vi "主界面B010.vi"() -> ()   [LabVIEW 2013]
uses:
  <vilib>/Utility/file.llb/Read From Spreadsheet File (string).vi
  PCI8622_32.dll
panel:
  out "是否检测轴承":dbl
  out "KSJS":string
  in  "Y挡圈最大值":dbl
  in  "Y挡圈最小值":dbl
  in  "X挡圈最大值":dbl
  in  "X挡圈最小值":dbl
  in  "Y内圈最大值":dbl
  in  "Y内圈最小值":dbl
  in  "X内圈最大值":dbl
  in  "X内圈最小值":dbl
  in  "Y轴承最大值":dbl
  in  "Y轴承最小值":dbl format="%#_13g"
  in  "X轴承最大值":dbl=12.0 format="%#_13g"
  in  "X轴承最小值":dbl=1.0 format="%#_13g"
  out "员工ID":string
  out "压铆最大压力(N)":dbl
  out "压铆最小压力(N)":dbl
  out "3最大压装位移":dbl
  out "3最小压装位移":dbl
  out "3监控点":dbl
  in  "压轴承换向压力":dbl=5000.0
  out "换向指示1":bool
  in  "报警工步号":dbl
  out "报警提示":string
  in  "轴承压头速度（手动）":dbl
  in  "轴承压头位置（手动）":dbl
  in  "轴承内圈压头速度（手动）":dbl
  in  "轴承内圈压头位置（手动）":dbl
  out "换向指示2":bool
  in  "换向压力2":dbl=5000.0
  in  "工步号复位":bool
  out "通讯状态":bool
  in  "电动缸2ARST":bool
  in  "电动缸1ARST":bool
  out "内圈压头位置(mm)":dbl format="%#.1f"
  out "轴承压头位置(mm)":dbl format="%#.1f"
  out "型号数量":i32
  out "轴承压头位移(mm)":dbl format="%#.1f"
  out "内圈位移(mm)":dbl format="%#.1f"
  out "压铆位移(mm)":dbl format="%#.1f"
  out "压铆压力(N)":dbl format="%#.1f"
  out "error out 4":errorcluster
  out "error out 3":errorcluster
  out "error out 2":errorcluster
  out "ADODB._Connection Out":refnum<k7>
  out "error out":errorcluster
  out "B010本序不合格":bool
  out "内圈压力(N)":dbl format="%#.1f"
  out "轴承压头压力(N)":dbl format="%#.1f"
  out "B010本序合格":bool
  in  "停止":bool
  in  "自动工步号":dbl
  out "产品选型":dbl
  out "芯片ID":string
  out "自动操作状态":string
  in  "联线按钮":bool
  in  "选项卡控件":T1(tab)
  out "轴承区域最小压力(N)":dbl
  out "轴承区域最大压力(N)":dbl
  out "压轴承最大压力(N)":dbl
  out "轴承压装位移(mm)":dbl
  out "轴承最小压装位移(mm)":dbl
  out "轴承最大压装位移(mm)":dbl
  out "轴承监控点":dbl
  out "压装轴承，挡圈曲线":cluster{"Y":dbl[], "Y":dbl[]}[](graph) caption="压球涨堵头1"
  out "轴承最小压力(N)":dbl
  out "轴承最大压力(N)":dbl
  out "压装轴承合格":bool
  out "压装轴承不合格":bool
  out "轴承监控点压力(N)":dbl
  out "内圈区域压力最大值(N)":dbl
  out "内圈区域压力最小值(N)":dbl
  out "内圈压装最大压力(N)":dbl
  out "压装滚针轴承":cluster{"Y":dbl[], "Y":dbl[]}[](graph) caption="压球涨堵头1"
  out "压内圈不合格":bool
  out "压内圈合格":bool
  out "内圈最大压力(N)":dbl
  out "内圈最小压力(N)":dbl
  out "内圈监控点":dbl
  out "内圈最大压装位移(mm)":dbl
  out "内圈最小压装位移(mm)":dbl
  out "内圈实测压装位移(mm)":dbl
  out "内圈监控点压力(N)":dbl
  out "压铆区域内最大压力(N)":dbl
  out "压铆区域内最小压力(N)":dbl
  out "挡圈压铆":cluster{"Y":dbl[], "Y":dbl[]}[](graph) caption="压球涨堵头1"
  out "压挡圈合格":bool
  out "压挡圈不合格":bool
  out "压铆最大压力(N)":dbl
  out "压铆压装位移(mm)":dbl
  in  "轴承单步":bool
  in  "内圈单步":bool
  in  "挡圈单步":bool
  out "轴承正面":bool
  in  "伺服2P 启动":bool
  in  "伺服1P 启动":bool
  in  "快速上升速度":dbl
  in  "快速上升位置":dbl
  in  "慢速下降速度":dbl
  in  "慢速下降位置":dbl
  in  "快速下降速度":dbl
  in  "快速下降位置":dbl
  in  "快速上升速度":dbl
  in  "快速上升位置":dbl
  in  "慢速下降速度":dbl
  in  "慢速下降位置":dbl
  in  "快速下降速度":dbl
  in  "伺服2回零":bool
  in  "伺服2上升":bool
  in  "伺服2下降":bool
  in  "伺服2复位":bool
  in  "快速下降位置":dbl
  in  "伺服1回零":bool
  in  "伺服1上升":bool
  in  "伺服1下降":bool
  in  "伺服1复位":bool
  out "急停按钮":bool
  out "联线状态":bool
  out "光幕保护":bool
  out "气压报警":bool
  out "滑台右位":bool
  out "滑台左位":bool
  in  "滑台右移":bool
  in  "滑台左移":bool
  in  "增压缸下压":bool
  in  "增压缸上升":bool
  in  "增压缸增压":bool
  in  "增压缸卸压":bool
  in  "压铆压力零点偏移":dbl format="%#.2f"
  in  "压铆压力比例偏移":dbl format="%#.2f"
  in  "压铆位移零点偏移":dbl format="%#.2f"
  in  "压铆位移比例偏移":dbl format="%#.2f"
  in  "内圈压力零点偏移":dbl format="%#.2f"
  in  "内圈压力比例偏移":dbl format="%#.2f"
  in  "内圈位移零点偏移":dbl format="%#.2f"
  in  "内圈位移比例偏移":dbl format="%#.2f"
  in  "轴承压力零点偏移":dbl format="%#.2f"
  in  "轴承压力比例偏移":dbl format="%#.2f"
  in  "轴承位移零点偏移":dbl format="%#.2f"
  in  "轴承位移比例偏移":dbl format="%#.2f"
  in  "传感器参数查询":bool
  in  "传感器参数保存":bool
  in  "参数浏览表":string[][](table)=[["J709", "J728", "J706"], ["1", "1", "1"], ["168", "78.5", "98"], ["0", "500", "500"], ["10000", "5000", "5000"], ["0", "78", "97"], ["173", "80", "102"], ["183", "85.5", "79"], ["0", "500", "500"], ["20000", "5000", "5000"], ["0", "85.5", "83"], ["190", "86.5", "84"], ["250", "144", "194"], ["0", "55000", "55000"], ["100000", "65000", "65000"], ["0", "143", "143"], ["300", "147", "147"], ["-70", "-89\n", "-94"], ["20", "50", "50"], ["-80.95", "-104", "-113"], ["1", "1", "1"], ["0", "0", "0"], ["20", "50", "50"], ["-77", "-70", "-75"], ["20", "50", "50"], ["-92.5", "-82", "-87"], ["1", "1", "1"], ["0", "0", "0"], ["20", "50", "50"], ["1", "95", "97"], ["84", "96", "99"], ["2000", "500", "500"], ["4000", "5000", "5000"], ["81", "75", "79"], ["82", "77", "81"], ["0", "500", "500"], ["25000", "5000", "5000"], ["250", "184", "193"], ["252", "186", "194"], ["10000", "10000", "10000"], ["60000", "50000", "50000"], ["", "5000", "5000"], ["", "5000", "5000"], ["", "93", "93"], ["", "100", "102"], ["", "-10", "-10"], ["", "10000", "10000"], ["", "71", "77"], ["", "80", "85"], ["", "-10", "-10"], ["", "6000", "6000"], ["", "180", "190"], ["", "190", "197"], ["", "-10", "-10"], ["", "70000", "70000"], ["", "0", "1"]]
  in  "参数查询":bool
  in  "试验参数保存":bool
  in  "轴承区域最小位移(mm)":dbl=84.0
  in  "轴承区域最大位移(mm)":dbl=85.0
  in  "轴承区域最小压力(N)":dbl=500.0
  in  "轴承区域最大压力(N)":dbl=5000.0
  in  "内圈区域最小位移(mm)":dbl=90.0
  in  "内圈区域最大位移(mm)":dbl=91.0
  in  "内圈区域最小压力(N)":dbl=500.0
  in  "内圈区域最大压力(N)":dbl=5000.0
  in  "挡圈区域最小位移(mm)":dbl=250.0
  in  "挡圈区域最大位移(mm)":dbl=252.0
  in  "挡圈区域最小压力(N)":dbl=10000.0
  in  "挡圈区域最大压力(N)":dbl=60000.0
  out "员工姓名":string
  in  "型号选择":u16(ring)=1 items=["J709", "J728", "J706"]
  in  "参数加载":bool
  out "产品ID":string="0"
  # "判定参数"
  # "芜湖机械转向器装配线"
  # "齿轮轴总成装配"
  # "Q14070机械转向器装配线"
  # "湖北唯思凌科装备制造有限公司 设计开发 (C)2015"
  # "判定参数"
  # "实测值"
  # "判定参数"
  # "实测值"
  # "实测值"
  # "轴承\n压头\n设置"
  # "轴承\n内圈\n压头\n设置"
  # "传感器校验区"
  # "注意：\n具备权限的用户才能够修改传感器校验参数和试验参数！"
  # "关于传感器校验：\n1、传感器校验需要由具备资质的单位或部门进行校验。\n2、具备权限的用户才能够修改传感器校验参数和试验参数。\n3、修改校验参数方法：先将比例偏移置为1，修改零点偏移，使零点值与校验的传感器一致；然后根据增幅调整比例偏移。"
  # "注意：\n具备权限的用户才能够修改传感器校验参数和试验参数！"
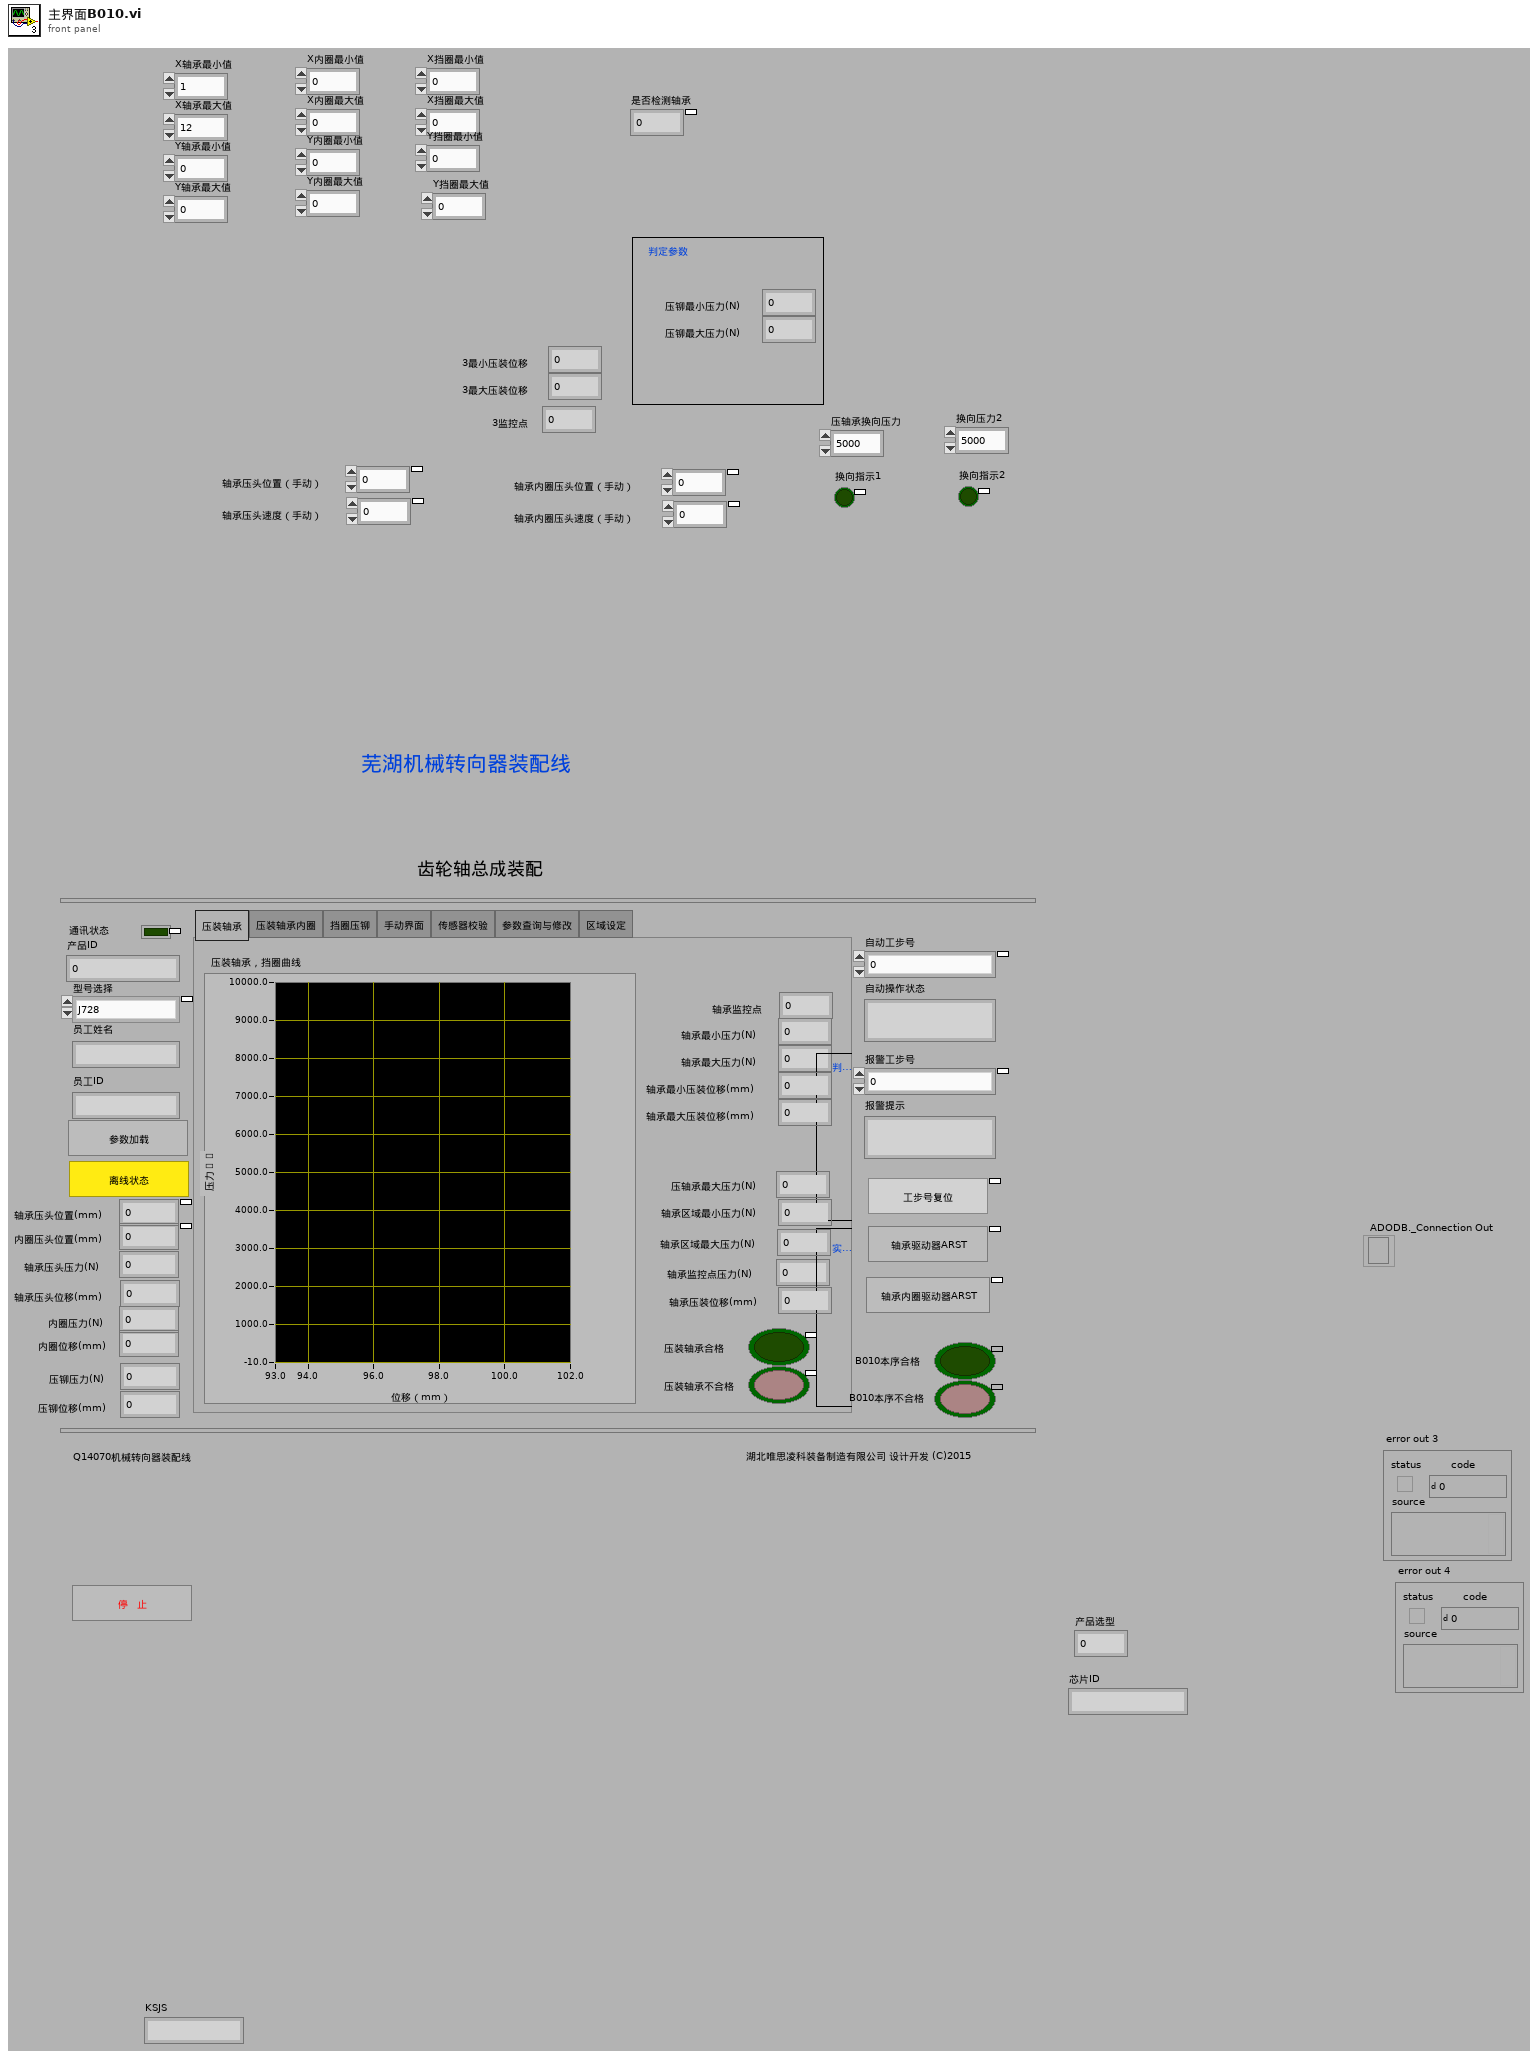
[diagram p1: front panel]
types:
  T1 = enum32{"压装轴承", "压装轴承内圈", "挡圈压铆", "手动界面", "传感器校验", "参数查询与修改", "区域设定"}
  T2 = typedef "imagedata.ctl" = cluster{"image type":i32, "image depth":i32, "image":u8[], "mask":u8[], "colors":u32[], "Rectangle":cluster{"left":i16, "top":i16, "right":i16, "bottom":i16}}
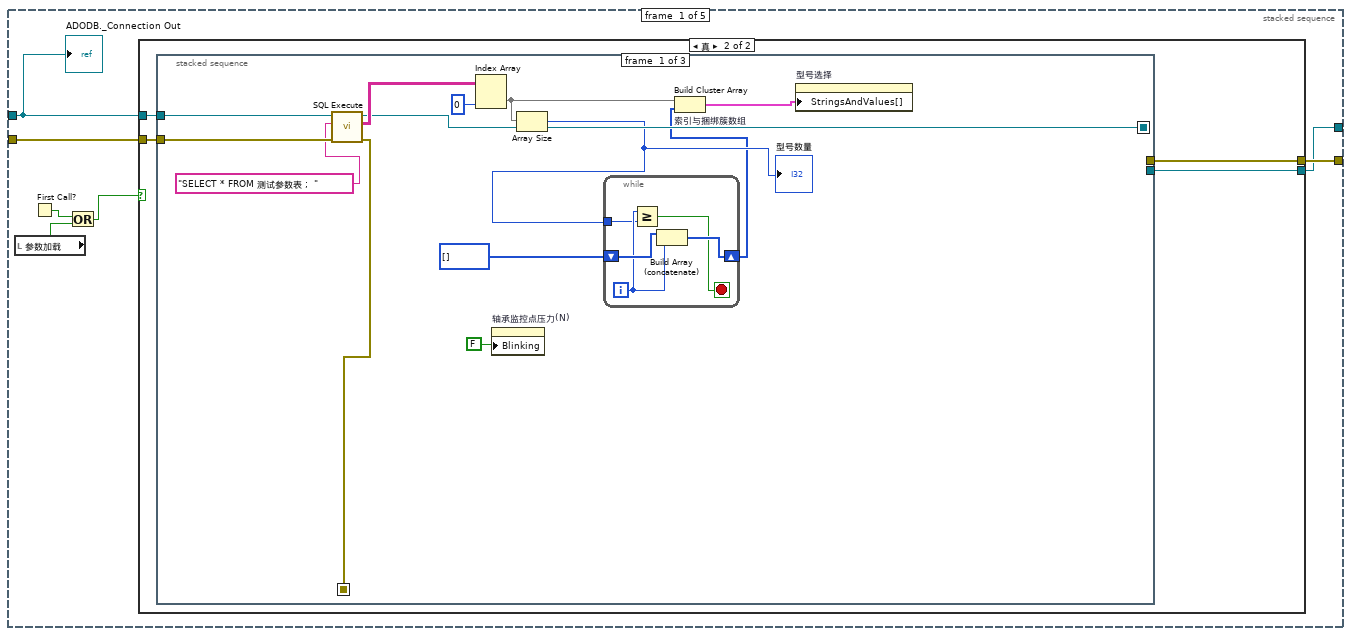
[diagram p2: hidden frame]
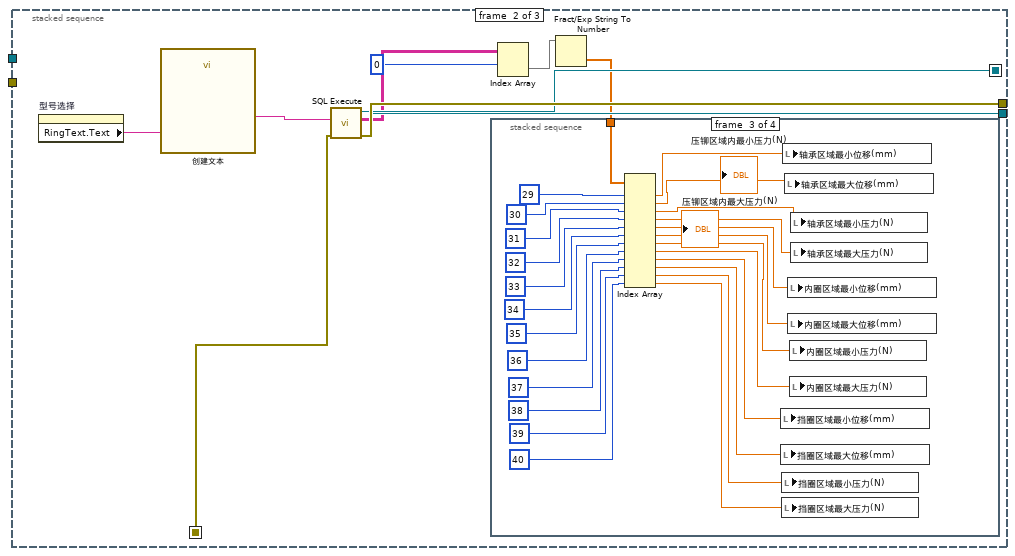
[diagram p4: hidden frame]
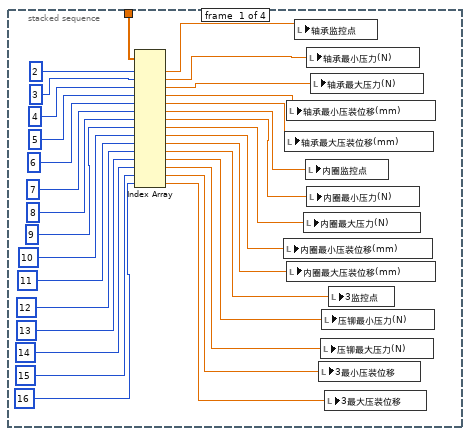
[diagram p5: hidden frame]
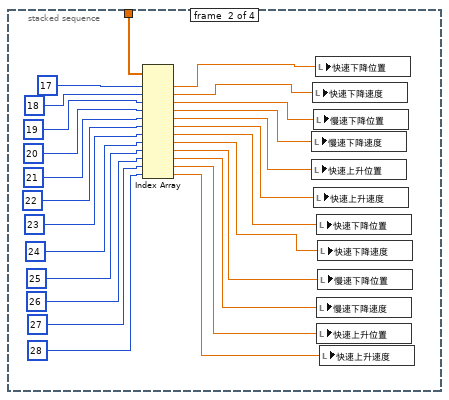
[diagram p6: hidden frame]
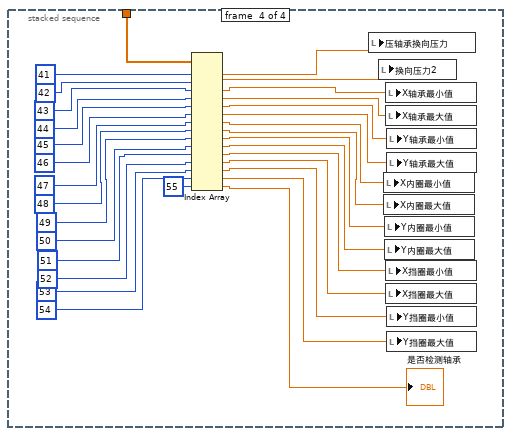
[diagram p7: hidden frame]
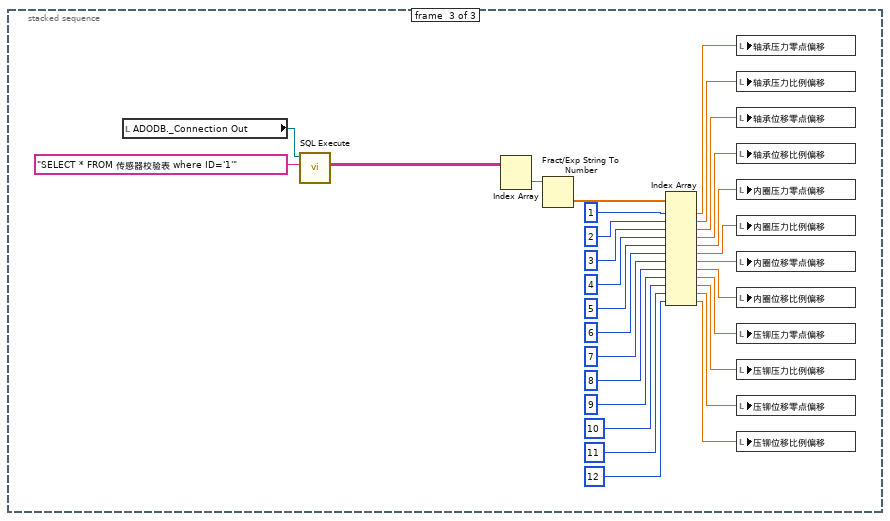
[diagram p8: hidden frame]
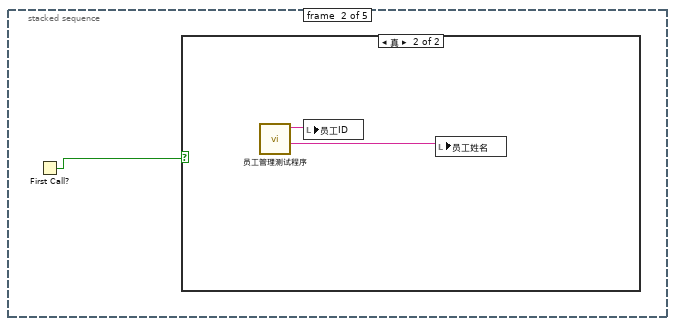
[diagram p9: hidden frame]
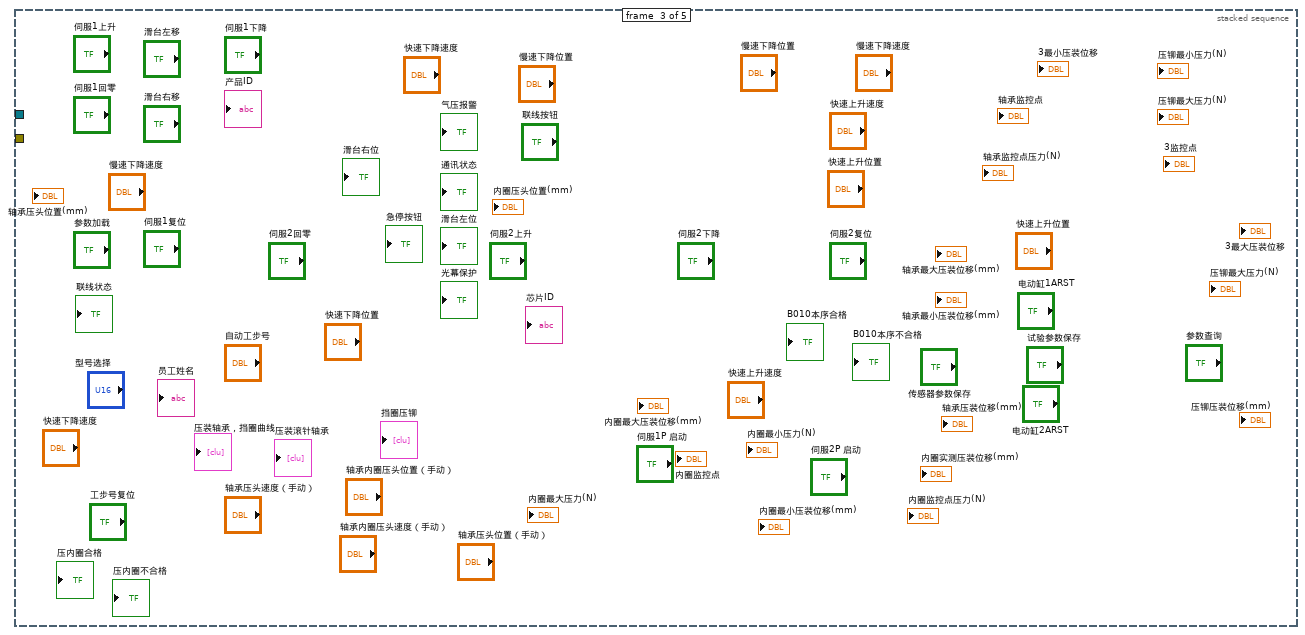
[diagram p11: hidden frame]
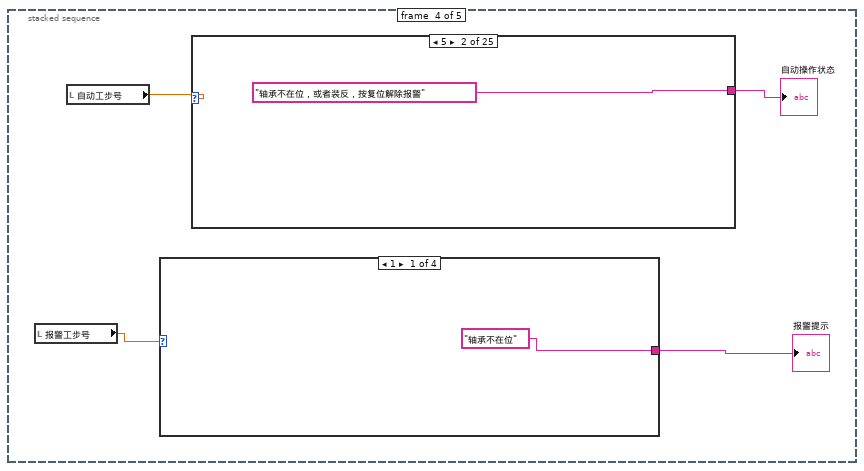
[diagram p12: hidden frame]
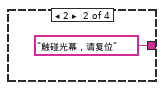
[diagram p13: hidden frame]
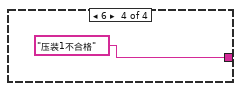
[diagram p15: hidden frame]
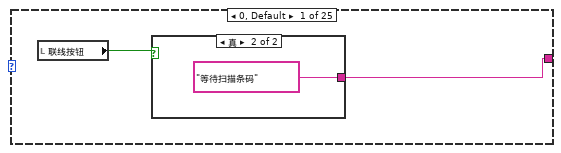
[diagram p16: hidden frame]
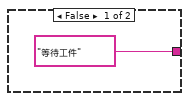
[diagram p17: hidden frame]
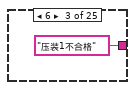
[diagram p18: hidden frame]
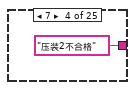
[diagram p19: hidden frame]
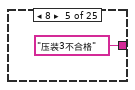
[diagram p20: hidden frame]
diagram:
  n1 = while {
    stop <- w10 stop-if-true
    n2 = local read "自动工步号"() -> (w8:dbl)
    n3 = Wait Until Next ms Multiple(millisecond multiple=u32 100 ("毫秒倍数")) -> ()  [unwired: 1 out]
    n4 = case shown="11" w8 {
      frame 0, Default {
      }
      frame 11 {
        n5 = flat-sequence {
          tunnel: [w27] -> w16
          tunnel: [w35] -> w22
          tunnel: [w34] -> w21
          tunnel: w16 -> [w33]
          tunnel: w22 -> [w61]
          tunnel: w21 -> [w59]
          tunnel: [w67] -> w20
          tunnel: [w66] -> w19
          tunnel: [w60] -> w14
          tunnel: w20 -> [w75]
          tunnel: w19 -> [w80]
          tunnel: [w77] -> w18
          tunnel: [w73] -> w17
          tunnel: [w72] -> w15
          tunnel: w14 -> [w72]
          tunnel: [w71] -> w13
          tunnel: [w70] -> w12
          tunnel: w18 -> [w89]
          tunnel: w17 -> [w88]
          tunnel: w15 -> [w85]
          tunnel: w13 -> [w87]
          tunnel: w12 -> [w86]
          tunnel: [w81] -> w11
          tunnel: w11 -> [w91]
          frame #0 {
            w25 = FALSE ("换向指示1")
            w32 = FALSE
            n6 = local write "压装轴承不合格"(w32) -> ()
            n7 = local write "压装轴承合格"(w32) -> ()
            n8 = Format Date/Time String(time format string (%c)="%Y%m%d%H%M%S" ("时间格式字符串(%c)")) -> (date/time string=→"KSJS":string)  [unwired: 2 in]
            n9 = property on="轴承监控点压力(N)" class="DigNum (严格)"("Blinking"=w25) -> ()  [unwired: 2 in, 2 out]
            n10 = local write "换向指示1"(w25) -> ()
            n11 = local write "换向指示2"(w25) -> ()
            n12 = local write "选项卡控件"(T1."压装轴承" ("选项卡控件")) -> ()
            n13 = call "区域曲线.vi"("区域最大压力(N)"="轴承区域最大压力(N)", "区域最小压力(N)"="轴承区域最小压力(N)", "区域最大位移(mm)"="轴承区域最大位移(mm)", "区域最小位移(mm)"="轴承区域最小位移(mm)") -> ("区域曲线"=w27:cluster{dbl[], dbl[]})  [unwired: 7 in]
          }
          frame #1 {
            w36 = dbl[] []
            n14 = while {
              shift-right: [w54] -> w35
              shift-left: w36 -> [w55]
              shift-right: [w52] -> w34
              shift-left: w36 -> [w53]
              tunnel: w33 -> [w42]
              stop <- w38 stop-if-true
              n15 = local read "轴承压头位置(mm)"() -> (w45:dbl)
              n16 = local read "自动工步号"() -> (w48:dbl)
              n17 = local read "轴承压头压力(N)"() -> (w51:dbl)
              n18 = local read "轴承压头压力(N)"() -> (w41:dbl)
              n19 = local read "压轴承换向压力"() -> (w40:dbl)
              n20 = Equal?(x=w48, y=30.0) -> (x = y?=w39:bool)
              n21 = Multiply(x=w45, y=-1.0) -> (x*y=w43:dbl)
              n22 = Build Array (concatenate)(w55, w43) -> (w54:dbl[])
              n23 = Build Array (concatenate)(w53, w51) -> (w52:dbl[])
              n24 = Bundle(w54, w52) -> (w50:cluster{dbl[], dbl[]})  [unwired: 1 in]
              n25 = Greater Or Equal?(x=w41, y=w40) -> (x >= y?=w37:bool)
              n26 = Build Array(w50, w42) -> (w49:cluster{dbl[], dbl[]}[])
              n27 = Or(x=w39, y=w37) -> (x .or. y?=w38:bool)
              n28 = local write "压装轴承，挡圈曲线"(w49) -> ()
              n29 = Wait Until Next ms Multiple(millisecond multiple=u32 50 ("毫秒倍数")) -> ()  [unwired: 1 out]
              n30 = local write "换向指示1"(w37) -> ()
            }
          }
          frame #2 {
            n31 = local read "轴承监控点"() -> (w69:dbl)
            n32 = local read "轴承区域最大位移(mm)"() -> (w64:dbl)
            n33 = local read "轴承区域最小位移(mm)"() -> (w65:dbl)
            n34 = local read "轴承区域最小压力(N)"() -> (w63:dbl)
            n35 = local read "轴承区域最大压力(N)"() -> (w62:dbl)
            n36 = Array Max & Min(array=w61) -> (max value=w66:dbl)  [unwired: 3 out]
            n37 = Array Max & Min(array=w59) -> (max value=→"压轴承最大压力(N)":dbl)  [unwired: 3 out]
            n38 = Threshold 1D Array "以阈值插值一维数组"(2:w69, 3:w61) -> (0:w68:dbl)  [unwired: 1 in]
            n39 = local write "轴承压装位移(mm)"(w66) -> ()
            n40 = Index Array(array=w59, index=w68) -> (element=w67:dbl)
            n41 = call "区域判断.vi"("压力数组"=w59, "位移数组"=w61, "区域最大压力"=w62, "区域最小压力"=w63, "区域最大位移"=w64, "区域最小位移"=w65) -> ("数值 2"=→"轴承区域最小压力(N)":dbl, "数值"=→"轴承区域最大压力(N)":dbl, "区域监控合格"=w60:bool)  [unwired: 1 in]
            n42 = local write "轴承监控点压力(N)"(w67) -> ()
          }
          frame #3 {
            n43 = local read "轴承最大压装位移(mm)"() -> (w79:dbl)
            n44 = local read "轴承最小压装位移(mm)"() -> (w78:dbl)
            n45 = local read "轴承最大压力(N)"() -> (w74:dbl)
            n46 = local read "轴承最小压力(N)"() -> (w76:dbl)
            n47 = In Range and Coerce(upper limit=w79, x=w80, lower limit=w78) -> (In Range?=w71:bool)  [unwired: 1 out]
            n48 = In Range and Coerce(upper limit=w74, x=w75, lower limit=w76) -> (In Range?=w70:bool)  [unwired: 1 out]
            n49 = Not(x=w71) -> (.not. x?=w77:bool)
            n50 = Not(x=w70) -> (.not. x?=w73:bool)
          }
          frame #4 {
            n51 = property on="轴承监控点压力(N)" class="DigNum (严格)"("Blinking"=w88) -> ()  [unwired: 2 in, 2 out]
            n52 = property on="轴承压装位移(mm)" class="DigNum (严格)"("Blinking"=w89) -> ()  [unwired: 2 in, 2 out]
            n53 = Compound Arithmetic op=AND(w87, w86, w85) -> (w84:bool)
            "压装轴承合格" <- w84
            n54 = Not(x=w84) -> (.not. x?=w83:bool)
            "压装轴承不合格" <- w83
            n55 = Wait Until Next ms Multiple(millisecond multiple=u32 80 ("毫秒倍数")) -> ()  [unwired: 1 out]
            n56 = local read "联线按钮"() -> (w82:bool)
            n57 = And(x=w83, y=w82) -> (x .and. y?=w81:bool)
          }
          frame #5 {
            n58 = case shown="真" w91 {
              frame False {
              }
              frame True {
                n59 = local write "B010本序不合格"(TRUE ("B010本序不合格")) -> ()
                n60 = local write "B010本序合格"(FALSE ("B010本序合格")) -> ()
              }
            }
          }
        }
      }
      frame 61 {
        n61 = flat-sequence {
          tunnel: [w109] -> w100
          tunnel: [w116] -> w106
          tunnel: [w115] -> w105
          tunnel: w100 -> [w114]
          tunnel: w106 -> [w142]
          tunnel: w105 -> [w140]
          tunnel: [w148] -> w104
          tunnel: [w147] -> w103
          tunnel: [w141] -> w98
          tunnel: w104 -> [w159]
          tunnel: w103 -> [w161]
          tunnel: [w160] -> w102
          tunnel: [w158] -> w101
          tunnel: [w153] -> w99
          tunnel: w98 -> [w153]
          tunnel: [w152] -> w97
          tunnel: [w151] -> w96
          tunnel: w102 -> [w169]
          tunnel: w101 -> [w168]
          tunnel: w99 -> [w167]
          tunnel: w97 -> [w166]
          tunnel: w96 -> [w165]
          tunnel: [w163] -> w95
          tunnel: [w162] -> w94
          tunnel: w95 -> [w173]
          tunnel: w94 -> [w172]
          frame #0 {
            w107 = FALSE
            n62 = property on="内圈监控点压力(N)" class="DigNum (严格)"("Blinking"=w107) -> ()  [unwired: 2 in, 2 out]
            n63 = local write "压内圈合格"(w107) -> ()
            n64 = local write "压内圈不合格"(w107) -> ()
            n65 = local write "换向指示2"(w107) -> ()
            n66 = local write "选项卡控件"(T1."压装轴承内圈" ("选项卡控件")) -> ()
            n67 = call "区域曲线.vi"("区域最大压力(N)"="内圈区域最大压力(N)", "区域最小压力(N)"="内圈区域最小压力(N)", "区域最大位移(mm)"="内圈区域最大位移(mm)", "区域最小位移(mm)"="内圈区域最小位移(mm)") -> ("区域曲线"=w109:cluster{dbl[], dbl[]})  [unwired: 7 in]
          }
          frame #1 {
            w117 = dbl[] []
            n68 = while {
              shift-right: [w135] -> w116
              shift-left: w117 -> [w136]
              shift-right: [w133] -> w115
              shift-left: w117 -> [w134]
              tunnel: w114 -> [w122]
              stop <- w121 stop-if-true
              n69 = local read "内圈压头位置(mm)"() -> (w124:dbl)
              n70 = local read "内圈压力(N)"() -> (w120:dbl)
              n71 = local read "内圈压力(N)"() -> (w123:dbl)
              n72 = local read "自动工步号"() -> (w131:dbl)
              n73 = Multiply(x=w124, y=-1.0) -> (x*y=w127:dbl)
              n74 = Build Array (concatenate)(w136, w127) -> (w135:dbl[])
              n75 = Build Array (concatenate)(w134, w123) -> (w133:dbl[])
              n76 = Equal?(x=w131, y=80.0) -> (x = y?=w129:bool)
              n77 = Greater Or Equal?(x=w120, y="换向压力2") -> (x >= y?=w118:bool)
              n78 = Or(x=w118, y=w129) -> (x .or. y?=w121:bool)
              n79 = Bundle(w135, w133) -> (w132:cluster{dbl[], dbl[]})  [unwired: 1 in]
              n80 = local write "换向指示2"(w118) -> ()
              n81 = Build Array(w132, w122) -> (w126:cluster{dbl[], dbl[]}[])
              n82 = local write "压装滚针轴承"(w126) -> ()
              n83 = Wait Until Next ms Multiple(millisecond multiple=u32 50 ("毫秒倍数")) -> ()  [unwired: 1 out]
            }
          }
          frame #2 {
            n84 = local read "内圈监控点"() -> (w149:dbl)
            n85 = local read "内圈区域最小位移(mm)"() -> (w146:dbl)
            n86 = local read "内圈区域最大位移(mm)"() -> (w145:dbl)
            n87 = local read "内圈区域最小压力(N)"() -> (w144:dbl)
            n88 = local read "内圈区域最大压力(N)"() -> (w143:dbl)
            n89 = Array Max & Min(array=w142) -> (max value=w147:dbl)  [unwired: 3 out]
            n90 = Array Max & Min(array=w140) -> (max value=→"内圈压装最大压力(N)":dbl)  [unwired: 3 out]
            n91 = Threshold 1D Array(2:w149, 3:w142) -> (0:w150:dbl)  [unwired: 1 in]
            n92 = Index Array(array=w140, index=w150) -> (element=w148:dbl)
            n93 = local write "内圈实测压装位移(mm)"(w147) -> ()
            n94 = local write "内圈监控点压力(N)"(w148) -> ()
            n95 = call "区域判断.vi"("压力数组"=w140, "位移数组"=w142, "区域最大压力"=w143, "区域最小压力"=w144, "区域最大位移"=w145, "区域最小位移"=w146) -> ("数值 2"=→"内圈区域压力最小值(N)":dbl, "数值"=→"内圈区域压力最大值(N)":dbl, "区域监控合格"=w141:bool)  [unwired: 1 in]
          }
          frame #3 {
            n96 = local read "内圈最大压装位移(mm)"() -> (w156:dbl)
            n97 = local read "内圈最小压装位移(mm)"() -> (w157:dbl)
            n98 = local read "内圈最小压力(N)"() -> (w154:dbl)
            n99 = local read "内圈最大压力(N)"() -> (w155:dbl)
            n100 = In Range and Coerce(upper limit=w156, x=w161, lower limit=w157) -> (In Range?=w152:bool)  [unwired: 1 out]
            n101 = In Range and Coerce(upper limit=w155, x=w159, lower limit=w154) -> (In Range?=w151:bool)  [unwired: 1 out]
            n102 = Not(x=w152) -> (.not. x?=w160:bool)
            n103 = Not(x=w151) -> (.not. x?=w158:bool)
          }
          frame #4 {
            n104 = property on="内圈监控点压力(N)" class="DigNum (严格)"("Blinking"=w168) -> ()  [unwired: 2 in, 2 out]
            n105 = property on="内圈实测压装位移(mm)" class="DigNum (严格)"("Blinking"=w169) -> ()  [unwired: 2 in, 2 out]
            n106 = Compound Arithmetic op=AND(w166, w167, w165) -> (w164:bool)
            n107 = Not(x=w164) -> (.not. x?=w163:bool)
            n108 = Wait Until Next ms Multiple(millisecond multiple=u32 80 ("毫秒倍数")) -> ()  [unwired: 1 out]
            n109 = local write "压内圈合格"(w164) -> ()
            n110 = local write "压内圈不合格"(w163) -> ()
            n111 = local read "联线按钮"() -> (w162:bool)
          }
          frame #5 {
            n112 = And(x=w173, y=w172) -> (x .and. y?=w171:bool)
            n113 = case shown="真" w171 {
              frame False {
              }
              frame True {
                n114 = local write "B010本序不合格"(TRUE ("B010本序不合格")) -> ()
                n115 = local write "B010本序合格"(FALSE ("B010本序合格")) -> ()
              }
            }
          }
        }
      }
      frame 110 {
        n116 = flat-sequence {
          tunnel: [w204] -> w192
          tunnel: [w196] -> w177
          tunnel: [w209] -> w195
          tunnel: [w208] -> w194
          tunnel: w192 -> [w207]
          tunnel: w177 -> [w206]
          tunnel: w195 -> [w229]
          tunnel: w194 -> [w230]
          tunnel: [w237] -> w185
          tunnel: [w238] -> w183
          tunnel: [w234] -> w181
          tunnel: [w233] -> w179
          tunnel: w185 -> [w244]
          tunnel: [w244] -> w184
          tunnel: w183 -> [w243]
          tunnel: [w243] -> w182
          tunnel: w181 -> [w242]
          tunnel: [w242] -> w180
          tunnel: w179 -> [w241]
          tunnel: [w241] -> w178
          tunnel: w184 -> [w257]
          tunnel: w182 -> [w259]
          tunnel: [w258] -> w193
          tunnel: w180 -> [w252]
          tunnel: [w252] -> w191
          tunnel: [w251] -> w190
          tunnel: [w250] -> w189
          tunnel: w178 -> [w247]
          tunnel: [w246] -> w186
          tunnel: [w245] -> w176
          tunnel: w193 -> [w268]
          tunnel: w191 -> [w262]
          tunnel: w190 -> [w263]
          tunnel: w189 -> [w267]
          tunnel: [w265] -> w188
          tunnel: [w264] -> w187
          tunnel: w186 -> [w261]
          tunnel: w176 -> [w260]
          tunnel: w188 -> [w272]
          tunnel: w187 -> [w271]
          frame #0 {
            w205 = FALSE
            n117 = local write "压挡圈不合格"(w205) -> ()
            n118 = local write "压挡圈合格"(w205) -> ()
            n119 = local write "选项卡控件"(T1."挡圈压铆" ("选项卡控件")) -> ()
            n120 = call "区域曲线.vi"("区域最大压力(N)"="挡圈区域最大压力(N)", "区域最小压力(N)"="挡圈区域最小压力(N)", "区域最大位移(mm)"="挡圈区域最大位移(mm)", "区域最小位移(mm)"="挡圈区域最小位移(mm)") -> ("区域曲线"=w204:cluster{dbl[], dbl[]})  [unwired: 7 in]
            n121 = call "区域曲线 - 副本.vi"("区域最大压力(N)"=100000.0, "区域最小压力(N)"=0.0, "区域最大位移(mm)"="挡圈区域最大位移(mm)", "区域最小位移(mm)"="挡圈区域最小位移(mm)") -> ("区域曲线1"=w196:cluster{dbl[], dbl[]})  [unwired: 7 in]
          }
          frame #1 {
            w210 = dbl[] []
            n122 = while {
              shift-right: [w213] -> w209
              shift-left: w210 -> [w225]
              shift-right: [w212] -> w208
              shift-left: w210 -> [w224]
              tunnel: w207 -> [w215]
              tunnel: w206 -> [w211]
              stop <- w220 stop-if-true
              n123 = local read "压铆压力(N)"() -> (w217:dbl)
              n124 = local read "压铆位移(mm)"() -> (w218:dbl)
              n125 = local read "自动工步号"() -> (w222:dbl)
              n126 = Build Array (concatenate)(w225, w218) -> (w213:dbl[])
              n127 = Build Array (concatenate)(w224, w217) -> (w212:dbl[])
              n128 = Equal?(x=w222, y=140.0) -> (x = y?=w220:bool)
              n129 = Bundle(w213, w212) -> (w223:cluster{dbl[], dbl[]})  [unwired: 1 in]
              n130 = Build Array(w223) -> (w216:cluster{dbl[], dbl[]}[])
              n131 = Build Array (concatenate)(w216, w215, w211) -> (w214:cluster{dbl[], dbl[]}[])
              n132 = Wait Until Next ms Multiple(millisecond multiple=u32 2 ("毫秒倍数")) -> ()  [unwired: 1 out]
              n133 = local write "挡圈压铆"(w214) -> ()
            }
          }
          frame #2 {
            n134 = local read "挡圈区域最小位移(mm)"() -> (w232:dbl)
            n135 = local read "挡圈区域最大位移(mm)"() -> (w231:dbl)
            n136 = local read "挡圈区域最大压力(N)"() -> (w235:dbl)
            n137 = local read "挡圈区域最小压力(N)"() -> (w236:dbl)
            n138 = local read "3监控点"() -> (w239:dbl)
            n139 = Array Max & Min(array=w229) -> (max value=w238:dbl)  [unwired: 3 out]
            n140 = Threshold 1D Array(2:w239, 3:w229) -> (0:w240:dbl)  [unwired: 1 in]
            n141 = Index Array(array=w230, index=w240) -> (element=w237:dbl)
            n142 = call "区域判断.vi"("压力数组"=w230, "位移数组"=w229, "区域最大压力"=w235, "区域最小压力"=w236, "区域最大位移"=w231, "区域最小位移"=w232) -> ("数值 2"=w228:dbl, "数值"=w227:dbl, "区域监控合格"=w234:bool)  [unwired: 1 in]
            n143 = local write "压铆压装位移(mm)"(w238) -> ()
            n144 = local write "压铆区域内最大压力(N)"(w227) -> ()
            n145 = local write "压铆区域内最小压力(N)"(w228) -> ()
            n146 = Array Max & Min(array=w230) -> (max value=w233:dbl)  [unwired: 3 out]
            n147 = local write "压铆最大压力(N)"(w233) -> ()
            n148 = property on="压铆最大压力(N)" class="DigNum (严格)"("Blinking"=FALSE ("闪烁")) -> ()  [unwired: 2 in, 2 out]
          }
          frame #3 {
          }
          frame #4 {
            n149 = local read "压铆最小压力(N)"() -> (w248:dbl)
            n150 = local read "挡圈区域最小压力(N)"() -> (w253:dbl)
            n151 = local read "压铆最大压力(N)"() -> (w249:dbl)
            n152 = local read "3最大压装位移"() -> (w256:dbl)
            n153 = local read "挡圈区域最大压力(N)"() -> (w254:dbl)
            n154 = local read "3最小压装位移"() -> (w255:dbl)
            n155 = In Range and Coerce(upper limit=w256, x=w259, lower limit=w255) -> (In Range?=w251:bool)  [unwired: 1 out]
            n156 = In Range and Coerce(upper limit=w254, x=w257, lower limit=w253) -> (In Range?=w250:bool)  [unwired: 1 out]
            n157 = In Range and Coerce(upper limit=w249, x=w247, lower limit=w248) -> (In Range?=w246:bool)  [unwired: 1 out]
            n158 = Not(x=w251) -> (.not. x?=w258:bool)
            n159 = Not(x=w246) -> (.not. x?=w245:bool)
          }
          frame #5 {
            n160 = property on="压铆最大压力(N)" class="DigNum (严格)"("Blinking"=w260) -> ()  [unwired: 2 in, 2 out]
            n161 = property on="压铆压装位移(mm)" class="DigNum (严格)"("Blinking"=w268) -> ()  [unwired: 2 in, 2 out]
            n162 = Compound Arithmetic op=AND(w267, w263, w262, w261) -> (w266:bool)
            n163 = Not(x=w266) -> (.not. x?=w265:bool)
            n164 = Wait Until Next ms Multiple(millisecond multiple=u32 80 ("毫秒倍数")) -> ()  [unwired: 1 out]
            n165 = local read "联线按钮"() -> (w264:bool)
            n166 = local write "压挡圈不合格"(w265) -> ()
            n167 = local write "压挡圈合格"(w266) -> ()
          }
          frame #6 {
            n168 = And(x=w272, y=w271) -> (x .and. y?=w270:bool)
            n169 = case shown="真" w270 {
              frame False {
              }
              frame True {
                n170 = local write "B010本序不合格"(TRUE ("B010本序不合格")) -> ()
                n171 = local write "B010本序合格"(FALSE ("B010本序合格")) -> ()
              }
            }
          }
        }
      }
      frame 150 {
        n172 = local read "联线按钮"() -> (w275:bool)
        n173 = case shown="真" w275 {
          frame False {
          }
          frame True {
            n174 = flat-sequence {
              tunnel: [w299] -> w276
              tunnel: w276 -> [w319]
              tunnel: ["F:\\报表储存\\"] -> w293
              tunnel: [w328] -> w292
              tunnel: [w327] -> w291
              tunnel: [w326] -> w290
              tunnel: [w325] -> w289
              tunnel: w293 -> [w355]
              tunnel: w292 -> [w354]
              tunnel: w291 -> [w353]
              tunnel: w290 -> [w352]
              tunnel: w289 -> [w341]
              tunnel: [w350] -> w288
              tunnel: [w349] -> w287
              tunnel: [w344] -> w286
              tunnel: [w343] -> w285
              tunnel: w288 -> [w359]
              tunnel: w287 -> [w358]
              tunnel: [w358] -> w284
              tunnel: w286 -> [w357]
              tunnel: [w357] -> w283
              tunnel: w285 -> [w356]
              tunnel: [w356] -> w282
              tunnel: w284 -> [w364]
              tunnel: w283 -> [w363]
              tunnel: [w363] -> w281
              tunnel: w282 -> [w362]
              tunnel: [w362] -> w280
              tunnel: w281 -> [w368]
              tunnel: [w368] -> w279
              tunnel: w280 -> [w367]
              tunnel: [w367] -> w278
              tunnel: w279 -> [w372]
              tunnel: w278 -> [w370]
              tunnel: [w370] -> w277
              tunnel: w277 -> [w378]
              frame #0 {
                n175 = Wait (ms)(milliseconds to wait=u32 500 ("毫秒倍数")) -> ()  [unwired: 1 out]
              }
              frame #1 {
                w297 = i16 3 ("宽度(-)")
                n176 = local read "压铆区域内最大压力(N)"() -> (w298:dbl)
                n177 = local read "员工ID"() -> (w317:string)
                n178 = local read "KSJS"() -> (w318:string)
                n179 = local read "轴承区域最小压力(N)"() -> (w314:dbl)
                n180 = local read "内圈压装最大压力(N)"() -> (w312:dbl)
                n181 = local read "轴承压装位移(mm)"() -> (w313:dbl)
                n182 = local read "压轴承最大压力(N)"() -> (w315:dbl)
                n183 = local read "压铆压装位移(mm)"() -> (w308:dbl)
                n184 = local read "内圈区域压力最小值(N)"() -> (w311:dbl)
                n185 = local read "内圈实测压装位移(mm)"() -> (w310:dbl)
                n186 = local read "压铆区域内最小压力(N)"() -> (w309:dbl)
                n187 = local read "压铆最大压力(N)"() -> (w296:dbl)
                n188 = Number To Fractional String(number=w315, precision (6)=w297) -> (F-format string=w316:string)  [unwired: 2 in]
                n189 = Number To Fractional String(number=w314, precision (6)=w297) -> (F-format string=w307:string)  [unwired: 2 in]
                n190 = Number To Fractional String(number=w313, precision (6)=w297) -> (F-format string=w306:string)  [unwired: 2 in]
                n191 = Number To Fractional String(number=w312, precision (6)=w297) -> (F-format string=w305:string)  [unwired: 2 in]
                n192 = Number To Fractional String(number=w309, precision (6)=w297) -> (F-format string=w301:string)  [unwired: 2 in]
                n193 = Number To Fractional String(number=w311, precision (6)=w297) -> (F-format string=w304:string)  [unwired: 2 in]
                n194 = Number To Fractional String(number=w296, precision (6)=w297) -> (F-format string=w295:string)  [unwired: 2 in]
                n195 = Number To Fractional String(number=w298, precision (6)=w297) -> (F-format string=w302:string)  [unwired: 2 in]
                n196 = Number To Fractional String(number=w308, precision (6)=w297) -> (F-format string=w300:string)  [unwired: 2 in]
                n197 = Number To Fractional String(number=w310, precision (6)=w297) -> (F-format string=w303:string)  [unwired: 2 in]
                n198 = Build Array(w318, w317, w316, w307, w306, w305, w304, w303, w302, w301, w300, w295) -> (w299:string[])
              }
              frame #2 {
                n199 = call "B010上传.vi"("数据"=w319) -> ()  [unwired: 3 in]
              }
              frame #3 {
                n200 = local read "产品ID"() -> (w323:string)
                n201 = Decimal String To Number(string=w323) -> (number=w322:i32)  [unwired: 2 in, 1 out]
                n202 = Wait (ms)(milliseconds to wait=u32 500 ("毫秒倍数")) -> ()  [unwired: 1 out]
                n203 = Increment(x=w322) -> (x+1=w321:i32)
                n204 = Number To Decimal String(number=w321) -> (decimal integer string=w320:string)  [unwired: 1 in]
                n205 = local write "产品ID"(w320) -> ()
              }
              frame #4 {
                n206 = local read "产品ID"() -> (w325:string)
                n207 = Format Date/Time String(time format string (%c)="%Y%m%d") -> (date/time string=w330:string)  [unwired: 2 in]
                n208 = String Subset(string=w330, offset (0)=6 ("偏移量(0)"), length (rest)=2 ("长度（剩余）")) -> (substring=w326:string)
                n209 = String Subset(string=w330, offset (0)=0 ("偏移量(0)"), length (rest)=4 ("长度（剩余）")) -> (substring=w328:string)
                n210 = String Subset(string=w330, offset (0)=4 ("偏移量(0)"), length (rest)=2 ("长度（剩余）")) -> (substring=w327:string)
              }
              frame #5 {
                w338 = "\\"
                n211 = Concatenate Strings(w355, w354, w338, w353, w338, w352, w338, w341, w338) -> (w351:string)
                n212 = Concatenate Strings(w355, w354, w338, w353, w338, w352, w338, w341, w338) -> (w342:string)
                n213 = String To Path(string=w351) -> (path=w350:path)
                n214 = Concatenate Strings(w342, w341, "轴承.JPG" ("字符串")) -> (w345:string)
                n215 = Concatenate Strings(w342, w341, "内圈.JPG" ("字符串")) -> (w346:string)
                n216 = Concatenate Strings(w342, w341, "挡圈.JPG" ("字符串")) -> (w348:string)
                n217 = String To Path(string=w345) -> (path=w343:path)
                n218 = String To Path(string=w346) -> (path=w344:path)
                n219 = String To Path(string=w348) -> (path=w349:path)
              }
              frame #6 {
                n220 = call <vilib>:"Check if File or Folder Exists.vi"("path"=w359) -> ("file or folder exists?"=w360:bool)  [unwired: 8 in, 2 out]
                n221 = case shown="假" w360 {
                  tunnel: w359 -> [w361 _]
                  frame False {
                    n222 = Create Folder(path (use dialog)=w361) -> ()  [unwired: 2 in, 3 out]
                  }
                  frame True {
                  }
                }
              }
              frame #7 {
                n223 = control-ref of="本VI"() -> (w366:refnum<vi>)
                n224 = invoke class="VI" method="FP.Get Image"(reference=w366) -> ("image data"=w365:T2)  [unwired: 5 in, 5 out]
                n225 = call <vilib>:"Write JPEG File.vi"("image data"=w365, "path to JPEG file"=w364) -> ()  [unwired: 8 in, 2 out]
              }
              frame #8 {
                n226 = Wait (ms)(milliseconds to wait=u32 500 ("毫秒倍数")) -> ()  [unwired: 1 out]
              }
              frame #9 {
                n227 = flat-sequence {
                  tunnel: w372 -> [w373]
                  tunnel: [w373] -> w371
                  tunnel: w371 -> [w376]
                  frame #0 {
                    n228 = local write "选项卡控件"(T1."压装轴承内圈" ("选项卡控件")) -> ()
                  }
                  frame #1 {
                    n229 = control-ref of="本VI"() -> (w377:refnum<vi>)
                    n230 = invoke class="VI" method="FP.Get Image"(reference=w377) -> ("image data"=w375:T2)  [unwired: 5 in, 5 out]
                    n231 = call <vilib>:"Write JPEG File.vi"("image data"=w375, "path to JPEG file"=w376) -> ()  [unwired: 8 in, 2 out]
                  }
                }
              }
              frame #10 {
                n232 = flat-sequence {
                  tunnel: w378 -> [w380]
                  frame #0 {
                    n233 = local write "选项卡控件"(T1."压装轴承" ("选项卡控件")) -> ()
                  }
                  frame #1 {
                    n234 = control-ref of="本VI"() -> (w382:refnum<vi>)
                    n235 = invoke class="VI" method="FP.Get Image"(reference=w382) -> ("image data"=w381:T2)  [unwired: 5 in, 5 out]
                    n236 = call <vilib>:"Write JPEG File.vi"("image data"=w381, "path to JPEG file"=w380) -> ()  [unwired: 8 in, 2 out]
                  }
                }
              }
              frame #11 {
                n237 = Wait (ms)(milliseconds to wait=u32 50 ("毫秒倍数")) -> ()  [unwired: 1 out]
                n238 = local write "选项卡控件"(T1."挡圈压铆" ("选项卡控件")) -> ()
              }
            }
          }
        }
      }
    }
    n239 = local read "停止"() -> (w10:bool)
  }
  n240 = while {
    stop <- w385 stop-if-true
    n241 = event shown="[6] \"试验参数保存\": 值改变" {
      selector: _ -> [_ _ _ _ _ _ _]
      dyn-events: _ -> [_ _ _ _ _ _ _]
      timeout: 500 -> [_ _ _ _ _ _ _]
      event Timeout {
        n242 = event-data() -> ()  [unwired: 3 out]
      }
      event "参数加载": Value Change {
        n243 = event-data() -> ()  [unwired: 7 out]
        n244 = property on="压装轴承，挡圈曲线" class="XYGraph (严格)"("YScale.Maximum"="Y轴承最大值") -> ()  [unwired: 2 in, 2 out]
        n245 = property on="压装轴承，挡圈曲线" class="XYGraph (严格)"("YScale.Minimum"="Y轴承最小值") -> ()  [unwired: 2 in, 2 out]
        n246 = property on="压装轴承，挡圈曲线" class="XYGraph (严格)"("XScale.Maximum"="X轴承最大值") -> ()  [unwired: 2 in, 2 out]
        n247 = property on="压装轴承，挡圈曲线" class="XYGraph (严格)"("XScale.Minimum"="X轴承最小值") -> ()  [unwired: 2 in, 2 out]
        n248 = property on="压装滚针轴承" class="XYGraph (严格)"("XScale.Maximum"="X内圈最大值") -> ()  [unwired: 2 in, 2 out]
        n249 = property on="压装滚针轴承" class="XYGraph (严格)"("XScale.Minimum"="X内圈最小值") -> ()  [unwired: 2 in, 2 out]
        n250 = property on="压装滚针轴承" class="XYGraph (严格)"("YScale.Maximum"="Y内圈最大值") -> ()  [unwired: 2 in, 2 out]
        n251 = property on="压装滚针轴承" class="XYGraph (严格)"("YScale.Minimum"="Y内圈最小值") -> ()  [unwired: 2 in, 2 out]
        n252 = property on="挡圈压铆" class="XYGraph (严格)"("XScale.Minimum"="X挡圈最小值") -> ()  [unwired: 2 in, 2 out]
        n253 = property on="挡圈压铆" class="XYGraph (严格)"("XScale.Maximum"="X挡圈最大值") -> ()  [unwired: 2 in, 2 out]
        n254 = property on="挡圈压铆" class="XYGraph (严格)"("YScale.Minimum"="Y挡圈最小值") -> ()  [unwired: 2 in, 2 out]
        n255 = property on="挡圈压铆" class="XYGraph (严格)"("YScale.Maximum"="Y挡圈最大值") -> ()  [unwired: 2 in, 2 out]
      }
      event "停止": Value Change {
        n256 = event-data() -> ()  [unwired: 7 out]
        n257 = flat-sequence {
          frame #0 {
          }
          frame #1 {
            n258 = Wait Until Next ms Multiple(millisecond multiple=u32 1000 ("毫秒倍数")) -> ()  [unwired: 1 out]
          }
          frame #2 {
            n259 = Quit LabVIEW(quit? (T)=TRUE ("停止？(T)")) -> ()
          }
        }
      }
      event "传感器参数查询": Value Change {
        n260 = event-data() -> ()  [unwired: 7 out]
        n261 = local read "ADODB._Connection Out"() -> (w419:refnum<k7>)
        n262 = call "SQL Execute.vi"("Command Text"="SELECT * FROM 传感器校验表 where ID='1'", "ADODB._Connection In"=w419) -> ("Data"=w420:string[][])  [unwired: 6 in, 3 out]
        n263 = Index Array(array=w420) -> (element=w421:string[])  [unwired: 2 in]
        n264 = Fract/Exp String To Number ("分数/指数字符串至数值转换")(string=w421) -> (number=w422:dbl[])  [unwired: 3 in, 1 out]
        n265 = Index Array(array=w422, index #1=1 ("索引"), index #2=2 ("索引"), index #3=3 ("索引"), index #4=4 ("索引"), index #5=5 ("索引"), index #6=6 ("索引"), index #7=7 ("索引"), index #8=8 ("索引"), index #9=9 ("索引"), index #10=10 ("索引"), index #11=11 ("索引"), index #12=12 ("索引")) -> (element #1=w427:dbl, element #2=w428:dbl, element #3=w429:dbl, element #4=w430:dbl, element #5=w409:dbl, element #6=w408:dbl, element #7=w407:dbl, element #8=w406:dbl, element #9=w405:dbl, element #10=w404:dbl, element #11=w403:dbl, element #12=w402:dbl)
        n266 = local write "轴承压力零点偏移"(w427) -> ()
        n267 = local write "轴承压力比例偏移"(w428) -> ()
        n268 = local write "轴承位移零点偏移"(w429) -> ()
        n269 = local write "轴承位移比例偏移"(w430) -> ()
        n270 = local write "内圈压力零点偏移"(w409) -> ()
        n271 = local write "内圈压力比例偏移"(w408) -> ()
        n272 = local write "内圈位移零点偏移"(w407) -> ()
        n273 = local write "内圈位移比例偏移"(w406) -> ()
        n274 = local write "压铆压力零点偏移"(w405) -> ()
        n275 = local write "压铆压力比例偏移"(w404) -> ()
        n276 = local write "压铆位移零点偏移"(w403) -> ()
        n277 = local write "压铆位移比例偏移"(w402) -> ()
      }
      event "参数查询": Value Change {
        n278 = event-data() -> ()  [unwired: 7 out]
        n279 = flat-sequence {
          tunnel: [w436] -> w431
          tunnel: [w441] -> w433
          tunnel: [w437] -> w432
          tunnel: w431 -> [w439]
          tunnel: w433 -> [w445]
          tunnel: w432 -> [w444]
          frame #0 {
            n280 = local read "ADODB._Connection Out"() -> (w436:refnum<k7>)
            n281 = call-poly <vilib>:"Read From Spreadsheet File.vi"("file path (dialog if empty)"=path "D:/Q14070-B010/参数/参数项.txt") -> ("first row"=w434:string[])  [unwired: 6 in, 4 out]
            n282 = property on="参数浏览表" class="Tbl (严格)"("Row Headers[]"=w434) -> ()  [unwired: 2 in, 2 out]
          }
          frame #1 {
            n283 = call "SQL Execute.vi"("Command Text"="SELECT * FROM 测试参数表;", "ADODB._Connection In"=w439) -> ("error out"=w441:errorcluster, "Data"=w442:string[][])  [unwired: 6 in, 2 out]
            n284 = Transpose 2D Array(2D array=w442) -> (transposed array=w437:string[][])
            n285 = Index Array(array=w437, index (row)=0 ("索引 (行)")) -> (element=w440:string[])  [unwired: 1 in]
            n286 = property on="参数浏览表" class="Tbl (严格)"("Column Headers[]"=w440) -> ()  [unwired: 2 in, 2 out]
          }
          frame #2 {
            n287 = local write "参数浏览表"(w444) -> ()
            "error out 2" <- w445
          }
        }
      }
      event "传感器参数保存": Value Change {
        n288 = event-data() -> ()  [unwired: 7 out]
        n289 = local read "轴承压力零点偏移"() -> (w484:dbl)
        n290 = local read "轴承压力比例偏移"() -> (w483:dbl)
        n291 = local read "轴承位移零点偏移"() -> (w482:dbl)
        n292 = local read "轴承位移比例偏移"() -> (w481:dbl)
        n293 = local read "内圈压力零点偏移"() -> (w480:dbl)
        n294 = local read "内圈压力比例偏移"() -> (w479:dbl)
        n295 = local read "内圈位移零点偏移"() -> (w478:dbl)
        n296 = local read "内圈位移比例偏移"() -> (w477:dbl)
        n297 = local read "压铆压力零点偏移"() -> (w476:dbl)
        n298 = local read "压铆压力比例偏移"() -> (w475:dbl)
        n299 = local read "压铆位移零点偏移"() -> (w474:dbl)
        n300 = local read "压铆位移比例偏移"() -> (w473:dbl)
        n301 = Build Array(w484, w483, w482, w481, w480, w479, w478, w477, w476, w475, w474, w473) -> (w472:dbl[])
        n302 = Number To Fractional String(number=w472, precision (6)=i16 2 ("精度(6)")) -> (F-format string=w470:string[])  [unwired: 2 in]
        n303 = Index Array(array=w470, index #1=0 ("索引"), index #2=1 ("索引"), index #3=2 ("索引"), index #4=3 ("索引"), index #5=4 ("索引"), index #6=5 ("索引"), index #7=6 ("索引"), index #8=7 ("索引"), index #9=8 ("索引"), index #10=9 ("索引"), index #11=10 ("索引"), index #12=11 ("索引")) -> (element #1=w457:string, element #2=w456:string, element #3=w455:string, element #4=w454:string, element #5=w453:string, element #6=w452:string, element #7=w451:string, element #8=w450:string, element #9=w449:string, element #10=w448:string, element #11=w447:string, element #12=w446:string)
        n304 = local read "ADODB._Connection Out"() -> (w485:refnum<k7>)
        n305 = call "创建文本3"("右压力零点偏移"=w457, "右压力比例偏移"=w456, "右位移零点偏移"=w455, "右位移比例偏移"=w454, "左压力零点偏移"=w453, "左压力比例偏移"=w452, "左位移零点偏移"=w451, "左位移比例偏移"=w450, "压铆压力零点偏移"=w449, "压铆压力比例偏移"=w448, "压铆位移零点偏移"=w447, "压铆位移比例偏移"=w446) -> ("Result"=w486:string)  [unwired: 14 in, 1 out]
        n306 = call "SQL Execute.vi"("Command Text"=w486, "ADODB._Connection In"=w485) -> ("error out"=w489:errorcluster, "ADODB._Connection Out"=w488:refnum<k7>)  [unwired: 6 in, 2 out]
        n307 = call "ADO Connection Close.vi"("error in (no error)"=w489, "ADODB._Connection In"=w488) -> ("error out"=→"error out 3":errorcluster)  [unwired: 8 in, 1 out]
      }
      event "试验参数保存": Value Change {
        n308 = event-data() -> ()  [unwired: 7 out]
        n309 = while {
          i -> [w494]
          stop <- w493 stop-if-true
          n310 = local read "型号数量"() -> (w491:i32)
          n311 = Wait Until Next ms Multiple(millisecond multiple=u32 50 ("毫秒倍数")) -> ()  [unwired: 1 out]
          n312 = Greater Or Equal?(x=w494, y=w491) -> (x >= y?=w493:bool)
          n313 = Index Array(array="参数浏览表", index (col)=w494) -> (element=w500:string[])  [unwired: 1 in]
          n314 = stacked-sequence "层叠式顺序结构" {
            seq-local: [w501 _ _ _] -> [_ w533 _ _]
            seq-local: [_ w535 _ _] -> [_ _ w565 _]
            seq-local: [_ _ w566 _] -> [_ _ _ w593]
            tunnel: w500 -> [w532 w536 w579 w625]
            tunnel: [_ _ _ w594] -> w490
            frame #0 {
              n315 = Index Array(array=w532, index #2=2 ("索引"), index #3=3 ("索引"), index #4=4 ("索引"), index #5=5 ("索引"), index #6=6 ("索引"), index #7=7 ("索引"), index #8=8 ("索引"), index #9=9 ("索引"), index #10=10 ("索引"), index #11=11 ("索引"), index #12=12 ("索引"), index #13=13 ("索引"), index #14=14 ("索引"), index #15=15 ("索引"), index #16=16 ("索引")) -> (element #2=w516:string, element #3=w515:string, element #4=w514:string, element #5=w513:string, element #6=w512:string, element #7=w511:string, element #8=w510:string, element #9=w509:string, element #10=w508:string, element #11=w507:string, element #12=w506:string, element #13=w505:string, element #14=w504:string, element #15=w503:string, element #16=w502:string)  [unwired: 1 in, 1 out]
              n316 = call "创建文本5"("1监控点"=w516, "1监控点最小压力"=w515, "1监控点最大压力"=w514, "1最小压装位移"=w513, "1最大压装位移"=w512, "2监控点"=w511, "2监控点最小压力"=w510, "2监控点最大压力"=w509, "2最小压装位移"=w508, "2最大压装位移"=w507, "3监控点"=w506, "3监控点最小压力"=w505, "3监控点最大压力"=w504, "3最小压装位移"=w503, "3最大压装位移"=w502) -> ("Result"=w501:string)  [unwired: 11 in, 1 out]
            }
            frame #1 {
              n317 = Index Array(array=w536, index #2=29 ("索引"), index #3=30 ("索引"), index #4=31 ("索引"), index #5=32 ("索引"), index #6=33 ("索引"), index #7=34 ("索引"), index #8=35 ("索引"), index #9=36 ("索引"), index #10=37 ("索引"), index #11=38 ("索引"), index #12=39 ("索引"), index #13=40 ("索引"), index #14=0 ("索引")) -> (element #2=w548:string, element #3=w547:string, element #4=w546:string, element #5=w545:string, element #6=w544:string, element #7=w543:string, element #8=w542:string, element #9=w541:string, element #10=w540:string, element #11=w539:string, element #12=w538:string, element #13=w537:string)  [unwired: 2 in, 3 out]
              n318 = call "创建文本2"("1区域最小位移"=w548, "1区域最大位移"=w547, "1区域最小压力"=w546, "1区域最大压力"=w545, "2区域最小位移"=w544, "2区域最大位移"=w543, "2区域最小压力"=w542, "2区域最大压力"=w541, "3区域最小位移"=w540, "3区域最大位移"=w539, "3区域最小压力"=w538, "3区域最大压力"=w537) -> ("Result"=w534:string)  [unwired: 14 in, 1 out]
              n319 = Concatenate Strings(w533, w534) -> (w535:string)
            }
            frame #2 {
              n320 = Index Array(array=w579, index #2=43 ("索引"), index #3=44 ("索引"), index #4=45 ("索引"), index #5=46 ("索引"), index #6=47 ("索引"), index #7=48 ("索引"), index #8=49 ("索引"), index #9=50 ("索引"), index #10=51 ("索引"), index #11=52 ("索引"), index #12=53 ("索引"), index #13=54 ("索引"), index #14=55 ("索引")) -> (element #2=w578:string, element #3=w577:string, element #4=w576:string, element #5=w575:string, element #6=w574:string, element #7=w573:string, element #8=w572:string, element #9=w571:string, element #10=w570:string, element #11=w569:string, element #12=w568:string, element #13=w567:string, element #14=w562:string)  [unwired: 2 in, 2 out]
              n321 = call "创建文本6"("X轴承最小值"=w578, "X轴承最大值"=w577, "Y轴承最小值"=w576, "Y轴承最大值"=w575, "X内圈最小值"=w574, "X内圈最大值"=w573, "Y内圈最小值"=w572, "Y内圈最大值"=w571, "X挡圈最小值"=w570, "X挡圈最大值"=w569, "Y挡圈最小值"=w568, "Y挡圈最大值"=w567, "是否检测轴承"=w562) -> ("Result"=w564:string)  [unwired: 13 in, 1 out]
              n322 = Concatenate Strings(w565, w564) -> (w566:string)
            }
            frame #3 {
              n323 = Index Array(array=w625, index #1=0 ("索引"), index #2=17 ("索引"), index #3=18 ("索引"), index #4=19 ("索引"), index #5=20 ("索引"), index #6=21 ("索引"), index #7=22 ("索引"), index #8=23 ("索引"), index #9=24 ("索引"), index #10=25 ("索引"), index #11=26 ("索引"), index #12=27 ("索引"), index #13=28 ("索引"), index #14=41 ("索引"), index #15=42 ("索引")) -> (element #1=w597:string, element #2=w611:string, element #3=w610:string, element #4=w609:string, element #5=w608:string, element #6=w607:string, element #7=w606:string, element #8=w605:string, element #9=w604:string, element #10=w603:string, element #11=w602:string, element #12=w601:string, element #13=w600:string, element #14=w596:string, element #15=w595:string)
              n324 = call "创建文本4"("1快下位置"=w611, "1快下速度"=w610, "1慢下位置"=w609, "1慢下速度"=w608, "1快上位置"=w607, "1快上速度"=w606, "2快下位置"=w605, "2快下速度"=w604, "2慢下位置"=w603, "2慢下速度"=w602, "2快上位置"=w601, "2快上速度"=w600, "压轴承换向力"=w596, "压内圈换向力"=w595, "产品型号"=w597) -> ("Result"=w592:string)  [unwired: 11 in, 1 out]
              n325 = Concatenate Strings(w593, w592) -> (w594:string)
            }
          }
          n326 = local read "ADODB._Connection Out"() -> (w492:refnum<k7>)
          n327 = call "SQL Execute.vi"("Command Text"=w490, "ADODB._Connection In"=w492) -> ("error out"=w498:errorcluster, "ADODB._Connection Out"=w499:refnum<k7>)  [unwired: 6 in, 2 out]
          n328 = call "ADO Connection Close.vi"("error in (no error)"=w498, "ADODB._Connection In"=w499) -> ("error out"=→"error out 4":errorcluster)  [unwired: 8 in, 1 out]
        }
      }
    }
    n329 = local read "停止"() -> (w385:bool)
    n330 = Wait Until Next ms Multiple(millisecond multiple=u32 50 ("毫秒倍数")) -> ()  [unwired: 1 out]
  }
  n331 = flat-sequence {
    tunnel: [w629] -> w4
    tunnel: [w627] -> w3
    tunnel: w4 -> [w634]
    tunnel: w3 -> [w633]
    tunnel: [w632] -> w2
    tunnel: [w631] -> w1
    tunnel: w2 -> [w867]
    tunnel: w1 -> [w866]
    frame #0 {
      n332 = call "ADO Connection Create.vi"() -> ("error out"=w628:errorcluster, "ADODB._Connection Out"=w630:refnum<k7>)  [unwired: 10 in]
      n333 = call "ADO Connection Open.vi"("error in (no error)"=w628, "ConnectionString"="Provider=Microsoft.Jet.OLEDB.4.0;Data Source=D:\\Q14070-B010\\参数\\参数B010.mdb;Persist Security Info=False;Jet OLEDB:Database Password=123;", "ADODB._Connection In"=w630) -> ("error out"=w627:errorcluster, "ADODB._Connection Out"=w629:refnum<k7>)  [unwired: 7 in]
    }
    frame #1 {
      n334 = while {
        tunnel: w634 -> [w638]
        tunnel: w633 -> [w637]
        tunnel: [w636] -> w632
        tunnel: [w635] -> w631
        stop <- w639 stop-if-true
        n335 = stacked-sequence {
          tunnel: w638 -> [w644 _ _ _ _]
          tunnel: w637 -> [w643 _ _ _ _]
          tunnel: [w641 _ _ _ _] -> w636
          tunnel: [w642 _ _ _ _] -> w635
          frame #0 {
            n336 = local read "参数加载"() -> (w646:bool)
            n337 = First Call?() -> (First Call?: T/F=w647:bool)
            n338 = Or(x=w647, y=w646) -> (x .or. y?=w645:bool)
            n339 = case shown="真" w645 {
              tunnel: w644 -> [_ w651]
              tunnel: w643 -> [_ w650]
              tunnel: [_ w649] -> w642
              tunnel: [_ w648] -> w641
              frame False {
              }
              frame True {
                n340 = stacked-sequence {
                  seq-local: [w658 _ _] -> [_ w679 _]
                  seq-local: [w657 _ _] -> [_ w677 _]
                  tunnel: w651 -> [w663 _ _]
                  tunnel: w650 -> [w660 _ _]
                  tunnel: [_ w678 _] -> w649
                  tunnel: [_ w676 _] -> w648
                  frame #0 {
                    n341 = call "SQL Execute.vi"("error in (no error)"=w660, "Command Text"="SELECT * FROM 测试参数表 ;  ", "ADODB._Connection In"=w663) -> ("error out"=w658:errorcluster, "Data"=w662:string[][], "ADODB._Connection Out"=w657:refnum<k7>)  [unwired: 5 in, 1 out]
                    n342 = Index Array(array=w662, index (col)=0 ("索引 (行)")) -> (element=w655:string[])  [unwired: 1 in]
                    n343 = property on="轴承监控点压力(N)" class="DigNum (严格)"("Blinking"=FALSE ("闪烁")) -> ()  [unwired: 2 in, 2 out]
                    n344 = Array Size(array=w655) -> (size(s)=w654:i32)
                    "型号数量" <- w654
                    n345 = while {
                      shift-right: [w669] -> w653
                      shift-left: i32[] [] -> [w668]
                      tunnel: w654 -> [w666]
                      i -> [w667]
                      stop <- w665 stop-if-true
                      n346 = Greater Or Equal?(x=w667, y=w666) -> (x >= y?=w665:bool)
                      n347 = Build Array (concatenate)(w668, w667) -> (w669:i32[])
                    }
                    n348 = Build Cluster Array "索引与捆绑簇数组"(w655, w653) -> (w661:cluster{"String":string, i32}[])
                    n349 = property on="型号选择" class="Ring (严格)"("StringsAndValues[]"=w661) -> ()  [unwired: 2 in, 2 out]
                  }
                  frame #1 {
                    n350 = property on="型号选择" class="Ring (严格)"() -> ("RingText.Text"=w674:string)  [unwired: 2 in, 2 out]
                    n351 = call "创建文本"("型号选择"=w674) -> ("Result"=w675:string)  [unwired: 13 in, 1 out]
                    n352 = call "SQL Execute.vi"("error in (no error)"=w679, "Command Text"=w675, "ADODB._Connection In"=w677) -> ("error out"=w678:errorcluster, "Data"=w673:string[][], "ADODB._Connection Out"=w676:refnum<k7>)  [unwired: 5 in, 1 out]
                    n353 = Index Array(array=w673, index (row)=0 ("索引 (行)")) -> (element=w671:string[])  [unwired: 1 in]
                    n354 = Fract/Exp String To Number ("分数/指数字符串至数值转换")(string=w671) -> (number=w670:dbl[])  [unwired: 3 in, 1 out]
                    n355 = stacked-sequence {
                      tunnel: w670 -> [w710 w735 w760 w791]
                      frame #0 {
                        n356 = Index Array ("索引数组")(array=w710, index #1=2 ("索引"), index #2=3 ("索引"), index #3=4 ("索引"), index #4=5 ("索引"), index #5=6 ("索引"), index #6=7 ("索引"), index #7=8 ("索引"), index #8=9 ("索引"), index #9=10 ("索引"), index #10=11 ("索引"), index #11=12 ("索引"), index #12=13 ("索引"), index #13=14 ("索引"), index #14=15 ("索引"), index #15=16 ("索引")) -> (element #1=w709:dbl, element #2=w708:dbl, element #3=w707:dbl, element #4=w706:dbl, element #5=w705:dbl, element #6=w704:dbl, element #7=w703:dbl, element #8=w702:dbl, element #9=w701:dbl, element #10=w700:dbl, element #11=w699:dbl, element #12=w698:dbl, element #13=w697:dbl, element #14=w696:dbl, element #15=w695:dbl)
                        n357 = local write "内圈最小压装位移(mm)"(w701) -> ()
                        n358 = local write "轴承最大压装位移(mm)"(w705) -> ()
                        n359 = local write "轴承最小压装位移(mm)"(w706) -> ()
                        n360 = local write "内圈最大压装位移(mm)"(w700) -> ()
                        n361 = local write "轴承监控点"(w709) -> ()
                        n362 = local write "内圈最大压力(N)"(w702) -> ()
                        n363 = local write "内圈监控点"(w704) -> ()
                        n364 = local write "轴承最小压力(N)"(w708) -> ()
                        n365 = local write "内圈最小压力(N)"(w703) -> ()
                        n366 = local write "轴承最大压力(N)"(w707) -> ()
                        n367 = local write "3最小压装位移"(w696) -> ()
                        n368 = local write "压铆最大压力(N)"(w697) -> ()
                        n369 = local write "压铆最小压力(N)"(w698) -> ()
                        n370 = local write "3最大压装位移"(w695) -> ()
                        n371 = local write "3监控点"(w699) -> ()
                      }
                      frame #1 {
                        n372 = Index Array(array=w735, index #1=17 ("索引"), index #2=18 ("索引"), index #3=19 ("索引"), index #4=20 ("索引"), index #5=21 ("索引"), index #6=22 ("索引"), index #7=23 ("索引"), index #8=24 ("索引"), index #9=25 ("索引"), index #10=26 ("索引"), index #11=27 ("索引"), index #12=28 ("索引")) -> (element #1=w722:dbl, element #2=w721:dbl, element #3=w720:dbl, element #4=w719:dbl, element #5=w718:dbl, element #6=w717:dbl, element #7=w716:dbl, element #8=w715:dbl, element #9=w714:dbl, element #10=w713:dbl, element #11=w712:dbl, element #12=w711:dbl)
                        n373 = local write "慢速下降速度"(w719) -> ()
                        n374 = local write "快速上升位置"(w718) -> ()
                        n375 = local write "快速下降速度"(w721) -> ()
                        n376 = local write "慢速下降位置"(w720) -> ()
                        n377 = local write "快速上升速度"(w717) -> ()
                        n378 = local write "快速下降位置"(w722) -> ()
                        n379 = local write "快速下降位置"(w716) -> ()
                        n380 = local write "慢速下降速度"(w713) -> ()
                        n381 = local write "快速上升位置"(w712) -> ()
                        n382 = local write "快速下降速度"(w715) -> ()
                        n383 = local write "慢速下降位置"(w714) -> ()
                        n384 = local write "快速上升速度"(w711) -> ()
                      }
                      frame #2 {
                        n385 = Index Array(array=w760, index #1=29 ("索引"), index #2=30 ("索引"), index #3=31 ("索引"), index #4=32 ("索引"), index #5=33 ("索引"), index #6=34 ("索引"), index #7=35 ("索引"), index #8=36 ("索引"), index #9=37 ("索引"), index #10=38 ("索引"), index #11=39 ("索引"), index #12=40 ("索引")) -> (element #1=w747:dbl, element #2=w746:dbl, element #3=w745:dbl, element #4=w744:dbl, element #5=w743:dbl, element #6=w742:dbl, element #7=w741:dbl, element #8=w740:dbl, element #9=w739:dbl, element #10=w738:dbl, element #11=w737:dbl, element #12=w736:dbl)
                        n386 = local write "挡圈区域最小位移(mm)"(w739) -> ()
                        n387 = local write "挡圈区域最大位移(mm)"(w738) -> ()
                        n388 = local write "挡圈区域最小压力(N)"(w737) -> ()
                        n389 = local write "挡圈区域最大压力(N)"(w736) -> ()
                        n390 = local write "轴承区域最小位移(mm)"(w747) -> ()
                        n391 = local write "轴承区域最大位移(mm)"(w746) -> ()
                        n392 = local write "内圈区域最小位移(mm)"(w743) -> ()
                        n393 = local write "内圈区域最大位移(mm)"(w742) -> ()
                        n394 = local write "内圈区域最小压力(N)"(w741) -> ()
                        n395 = local write "内圈区域最大压力(N)"(w740) -> ()
                        n396 = local write "轴承区域最小压力(N)"(w745) -> ()
                        n397 = local write "轴承区域最大压力(N)"(w744) -> ()
                      }
                      frame #3 {
                        n398 = Index Array(array=w791, index #1=41 ("索引"), index #2=42 ("索引"), index #3=43 ("索引"), index #4=44 ("索引"), index #5=45 ("索引"), index #6=46 ("索引"), index #7=47 ("索引"), index #8=48 ("索引"), index #9=49 ("索引"), index #10=50 ("索引"), index #11=51 ("索引"), index #12=52 ("索引"), index #13=53 ("索引"), index #14=54 ("索引"), index #15=55 ("索引")) -> (element #1=w787:dbl, element #2=w788:dbl, element #3=w774:dbl, element #4=w773:dbl, element #5=w772:dbl, element #6=w771:dbl, element #7=w770:dbl, element #8=w769:dbl, element #9=w768:dbl, element #10=w767:dbl, element #11=w766:dbl, element #12=w765:dbl, element #13=w764:dbl, element #14=w763:dbl, element #15=→"是否检测轴承":dbl)
                        n399 = local write "压轴承换向压力"(w787) -> ()
                        n400 = local write "换向压力2"(w788) -> ()
                        n401 = local write "X内圈最小值"(w770) -> ()
                        n402 = local write "X内圈最大值"(w769) -> ()
                        n403 = local write "Y内圈最小值"(w768) -> ()
                        n404 = local write "Y内圈最大值"(w767) -> ()
                        n405 = local write "X轴承最小值"(w774) -> ()
                        n406 = local write "X轴承最大值"(w773) -> ()
                        n407 = local write "X挡圈最小值"(w766) -> ()
                        n408 = local write "X挡圈最大值"(w765) -> ()
                        n409 = local write "Y轴承最小值"(w772) -> ()
                        n410 = local write "Y轴承最大值"(w771) -> ()
                        n411 = local write "Y挡圈最小值"(w764) -> ()
                        n412 = local write "Y挡圈最大值"(w763) -> ()
                      }
                    }
                  }
                  frame #2 {
                    n413 = local read "ADODB._Connection Out"() -> (w809:refnum<k7>)
                    n414 = call "SQL Execute.vi"("Command Text"="SELECT * FROM 传感器校验表 where ID='1'", "ADODB._Connection In"=w809) -> ("Data"=w810:string[][])  [unwired: 6 in, 3 out]
                    n415 = Index Array(array=w810) -> (element=w811:string[])  [unwired: 2 in]
                    n416 = Fract/Exp String To Number ("分数/指数字符串至数值转换")(string=w811) -> (number=w812:dbl[])  [unwired: 3 in, 1 out]
                    n417 = Index Array(array=w812, index #1=1 ("索引"), index #2=2 ("索引"), index #3=3 ("索引"), index #4=4 ("索引"), index #5=5 ("索引"), index #6=6 ("索引"), index #7=7 ("索引"), index #8=8 ("索引"), index #9=9 ("索引"), index #10=10 ("索引"), index #11=11 ("索引"), index #12=12 ("索引")) -> (element #1=w817:dbl, element #2=w818:dbl, element #3=w819:dbl, element #4=w820:dbl, element #5=w799:dbl, element #6=w798:dbl, element #7=w797:dbl, element #8=w796:dbl, element #9=w795:dbl, element #10=w794:dbl, element #11=w793:dbl, element #12=w792:dbl)
                    n418 = local write "轴承压力零点偏移"(w817) -> ()
                    n419 = local write "轴承压力比例偏移"(w818) -> ()
                    n420 = local write "轴承位移零点偏移"(w819) -> ()
                    n421 = local write "轴承位移比例偏移"(w820) -> ()
                    n422 = local write "内圈压力零点偏移"(w799) -> ()
                    n423 = local write "内圈压力比例偏移"(w798) -> ()
                    n424 = local write "内圈位移零点偏移"(w797) -> ()
                    n425 = local write "内圈位移比例偏移"(w796) -> ()
                    n426 = local write "压铆压力零点偏移"(w795) -> ()
                    n427 = local write "压铆压力比例偏移"(w794) -> ()
                    n428 = local write "压铆位移零点偏移"(w793) -> ()
                    n429 = local write "压铆位移比例偏移"(w792) -> ()
                  }
                }
              }
            }
            "ADODB._Connection Out" <- w644
          }
          frame #1 {
            n430 = First Call?() -> (First Call?: T/F=w821:bool)
            n431 = case shown="真" w821 {
              frame False {
              }
              frame True {
                n432 = call "员工管理测试程序.vi"() -> ("员工姓名"=w823:string, "员工ID"=w822:string)  [unwired: 10 in]
                n433 = local write "员工ID"(w822) -> ()
                n434 = local write "员工姓名"(w823) -> ()
              }
            }
          }
          frame #2 {
          }
          frame #3 {
            n435 = local read "报警工步号"() -> (w825:dbl)
            n436 = local read "自动工步号"() -> (w827:dbl)
            n437 = case shown="1" w825 {
              tunnel: ["轴承不在位" ("工步操作状态") "触碰光幕，请复位" ("工步操作状态") _ "压装1不合格" ("工步操作状态")] -> w824
              frame 1 {
              }
              frame 2 {
              }
              frame 0, Default {
              }
              frame 6 {
              }
            }
            "报警提示" <- w824
            n438 = case shown="5" w827 {
              tunnel: [w831 "轴承不在位，或者装反，按复位解除报警" ("工步操作状态") "压装1不合格" ("工步操作状态") "压装2不合格" ("工步操作状态") "压装3不合格" ("工步操作状态") "请释放急停按钮" ("工步操作状态") "伺服1快下" ("工步操作状态") "伺服1慢下" ("工步操作状态") "保压中" ("工步操作状态") "伺服1快速上升" ("工步操作状态") "滑台左移" ("工步操作状态") "伺服2快下" ("工步操作状态") "伺服2慢下" ("工步操作状态") "伺服2慢下" ("工步操作状态") "保压中" ("工步操作状态") "伺服2快速上升" ("工步操作状态") "压铆启动" ("工步操作状态") "等待开始增压" ("工步操作状态") "保压" ("工步操作状态") "泄压" ("工步操作状态") "压铆上升，右移" ("工步操作状态") "请取挡圈" ("工步操作状态") "涂脂" ("工步操作状态") "压装不合格" ("工步操作状态") "数据上传完成" ("工步操作状态")] -> w826
              frame 0, Default {
                n439 = local read "联线按钮"() -> (w832:bool)
                n440 = case shown="真" w832 {
                  tunnel: ["等待工件" ("工步操作状态") "等待扫描条码" ("工步操作状态")] -> w831
                  frame False {
                  }
                  frame True {
                  }
                }
              }
              frame 5 {
              }
              frame 6 {
              }
              frame 7 {
              }
              frame 8 {
              }
              frame 9 {
              }
              frame 10 {
              }
              frame 20 {
              }
              frame 30 {
              }
              frame 40 {
              }
              frame 50 {
              }
              frame 60 {
              }
              frame 65 {
              }
              frame 70 {
              }
              frame 80 {
              }
              frame 90 {
              }
              frame 100 {
              }
              frame 120 {
              }
              frame 130 {
              }
              frame 140 {
              }
              frame 150 {
              }
              frame 170 {
              }
              frame 180 {
              }
              frame 800 {
              }
              frame 900 {
              }
            }
            "自动操作状态" <- w826
          }
          frame #4 {
            n441 = flat-sequence {
              frame #0 {
                n442 = First Call?() -> (First Call?: T/F=w859:bool)
                n443 = case shown="真" w859 {
                  frame False {
                  }
                  frame True {
                    n444 = local write "B010本序不合格"(FALSE ("B010本序不合格")) -> ()
                    n445 = local write "B010本序合格"(TRUE ("B010本序合格")) -> ()
                  }
                }
              }
              frame #1 {
                n446 = while {
                  stop <- w863 stop-if-true
                  n447 = local read "B010本序不合格"() -> (w862:bool)
                  n448 = case shown="真" w862 {
                    frame False {
                    }
                    frame True {
                      n449 = call "显示对话框信息"() -> ()  [unwired: 10 in, 2 out]
                    }
                  }
                  n450 = local read "B010本序合格"() -> (w863:bool)
                  n451 = Wait Until Next ms Multiple(millisecond multiple=u32 50 ("毫秒倍数")) -> ()  [unwired: 1 out]
                }
              }
            }
          }
        }
        n452 = Wait Until Next ms Multiple(millisecond multiple=u32 50 ("毫秒倍数")) -> ()  [unwired: 1 out]
        n453 = local read "停止"() -> (w639:bool)
      }
    }
    frame #2 {
      n454 = call "ADO Connection Close.vi"("error in (no error)"=w866, "ADODB._Connection In"=w867) -> ("error out"=→"error out":errorcluster)  [unwired: 8 in, 1 out]
    }
  }
  n455 = flat-sequence {
    tunnel: [w868] -> w7
    tunnel: w7 -> [w870]
    tunnel: [w869] -> w6
    tunnel: w6 -> [w958]
    tunnel: [w958] -> w5
    tunnel: w5 -> [w960]
    frame #0 {
      n456 = call "PCI8622配置.vi"() -> ("DeviceID"=w868:i32)  [unwired: 11 in]
    }
    frame #1 {
      n457 = while {
        tunnel: w870 -> [w945]
        tunnel: [w945] -> w869
        stop <- "停止" stop-if-true
        w955 = 0  # nRetSizeWords
        w956 = 2048  # nReadSizeWords
        # "hDevice"
        n458 = Wait Until Next ms Multiple(millisecond multiple=u32 50 ("毫秒倍数")) -> ()  [unwired: 1 out]
        n459 = Initialize Array(u16 0, 2048 ("dimension size")) -> (w946:u16[])
        n460 = dll-call lib="PCI8622_32.dll" fn="PCI8622_ReadDeviceProAD_Npt" label="ReadDeviceProAD_Npt"("hDevice"=w945, "ADBuffer[]"=w946, "nReadSizeWords"=w956, "nRetSizeWords"=w955) -> ("ADBuffer[]"=w949:u16[])  [unwired: 7 in, 2 out]
        n461 = Divide(x=w949, y=65536.01) -> (x/y=w950:dbl[])
        n462 = Multiply(x=w950, y=20) -> (x*y=w953:dbl[])
        n463 = Subtract(x=w953, y=10) -> (x-y=w934:dbl[])
        n464 = Decimate 1D Array "抽取一维数组"(w934) -> (w936:dbl[], w935:dbl[], w942:dbl[], w931:dbl[], w919:dbl[], w918:dbl[])  [unwired: 2 out]
        n465 = Add Array Elements(numeric array=w936) -> (sum=w937:dbl)
        n466 = Add Array Elements(numeric array=w935) -> (sum=w939:dbl)
        n467 = Add Array Elements(numeric array=w942) -> (sum=w943:dbl)
        n468 = Add Array Elements(numeric array=w931) -> (sum=w933:dbl)
        n469 = Array Size(array=w936) -> (size(s)=w938:i32)
        n470 = Array Size(array=w935) -> (size(s)=w940:i32)
        n471 = Array Size(array=w942) -> (size(s)=w941:i32)
        n472 = Array Size(array=w931) -> (size(s)=w932:i32)
        n473 = Add Array Elements(numeric array=w919) -> (sum=w924:dbl)
        n474 = Add Array Elements(numeric array=w918) -> (sum=w922:dbl)
        n475 = Array Size(array=w919) -> (size(s)=w923:i32)
        n476 = Array Size(array=w918) -> (size(s)=w921:i32)
        n477 = Divide(x=w937, y=w938) -> (x/y=w910:dbl)
        n478 = Divide(x=w939, y=w940) -> (x/y=w890:dbl)
        n479 = Divide(x=w943, y=w941) -> (x/y=w892:dbl)
        n480 = Divide(x=w933, y=w932) -> (x/y=w888:dbl)
        n481 = Divide(x=w924, y=w923) -> (x/y=w886:dbl)
        n482 = Divide(x=w922, y=w921) -> (x/y=w883:dbl)
        n483 = local read "内圈压力零点偏移"() -> (w878:dbl)
        n484 = Multiply(x=w883, y=30.0) -> (x*y=w882:dbl)
        n485 = Multiply(x=w888, y=30.0) -> (x*y=w899:dbl)
        n486 = Multiply(x=w892, y=-10000.0) -> (x*y=w902:dbl)
        n487 = local read "压铆压力零点偏移"() -> (w876:dbl)
        n488 = Multiply(x=w910, y=2000.0) -> (x*y=w908:dbl)
        n489 = local read "轴承压力零点偏移"() -> (w926:dbl)
        n490 = local read "压铆位移零点偏移"() -> (w874:dbl)
        n491 = local read "内圈位移零点偏移"() -> (w880:dbl)
        n492 = Multiply(x=w886, y=30.0) -> (x*y=w885:dbl)
        n493 = Multiply(x=w890, y=500.0) -> (x*y=w905:dbl)
        n494 = Subtract(x=w882, y=0.0) -> (x-y=w881:dbl)
        n495 = local read "轴承位移零点偏移"() -> (w872:dbl)
        n496 = Subtract(x=w899, y=0.0) -> (x-y=w887:dbl)
        n497 = Subtract(x=w902, y=90.6) -> (x-y=w891:dbl)
        n498 = Subtract(x=w908, y=515.3) -> (x-y=w893:dbl)
        n499 = local read "压铆压力比例偏移"() -> (w875:dbl)
        n500 = Subtract(x=w885, y=0.0) -> (x-y=w884:dbl)
        n501 = local read "轴承压力比例偏移"() -> (w925:dbl)
        n502 = local read "内圈位移比例偏移"() -> (w879:dbl)
        n503 = local read "轴承位移比例偏移"() -> (w871:dbl)
        n504 = Subtract(x=w905, y=256.8) -> (x-y=w889:dbl)
        n505 = local read "压铆位移比例偏移"() -> (w873:dbl)
        n506 = local read "内圈压力比例偏移"() -> (w877:dbl)
        n507 = Subtract(x=w891, y=w876) -> (x-y=w920:dbl)
        n508 = Subtract(x=w889, y=w878) -> (x-y=w928:dbl)
        n509 = Subtract(x=w884, y=w880) -> (x-y=w916:dbl)
        n510 = Subtract(x=w887, y=w874) -> (x-y=w917:dbl)
        n511 = Subtract(x=w893, y=w926) -> (x-y=w930:dbl)
        n512 = Subtract(x=w881, y=w872) -> (x-y=w915:dbl)
        n513 = Multiply(x=w920, y=w875) -> (x*y=→"压铆压力(N)":dbl)
        n514 = Multiply(x=w930, y=w925) -> (x*y=→"轴承压头压力(N)":dbl)
        n515 = Multiply(x=w928, y=w877) -> (x*y=→"内圈压力(N)":dbl)
        n516 = Multiply(x=w917, y=w873) -> (x*y=→"压铆位移(mm)":dbl)
        n517 = Multiply(x=w916, y=w879) -> (x*y=→"内圈位移(mm)":dbl)
        n518 = Multiply(x=w915, y=w871) -> (x*y=→"轴承压头位移(mm)":dbl)
      }
    }
    frame #2 {
      n519 = dll-call lib="PCI8622_32.dll" fn="PCI8622_StopDeviceProAD" label="StopDeviceProAD"("hDevice"=w958) -> ("hDevice"=w959:i32)  [unwired: 4 in, 2 out]
      n520 = dll-call lib="PCI8622_32.dll" fn="PCI8622_ReleaseDeviceProAD" label="ReleaseDeviceProAD"("hDevice"=w959) -> ()  [unwired: 5 in, 2 out]
    }
    frame #3 {
      n521 = dll-call lib="PCI8622_32.dll" fn="PCI8622_ReleaseDevice" label="ReleaseDevice"("hDevice"=w960) -> ()  [unwired: 5 in, 2 out]
    }
  }
